vi "02Config_equipos.vi"(4 "EE 568 M IN":T2(array[cluster]) {"Analogicas 32"."?" items=["1", "2", "4", "8", "16", "32", "64", "128", "256"]; "Analogicas 32"."?" items=["Lineal"=15, "Cuadrática"=14]; "Analogicas 32"."unsigned byte array[0]" items=["10000", "1000", "100", "10", "8000", "800", "80", "8", "4000", "400", "40", "4", "2000", "200", "20", "2"]; "Analogicas 16"."?" items=["1", "2", "4", "8", "16", "32", "64", "128", "256"]; "Analogicas 16"."?" items=["Lineal"=15, "Cuadrática"=14]; "Analogicas 16"."unsigned byte array[0]" items=["10000", "1000", "100", "10", "8000", "800", "80", "8", "4000", "400", "40", "4", "2000", "200", "20", "2"]}, 6 "Equipo Nº":i32(ring) caption="PANEL DE EQUIPO\nA CONFIGURAR" items=["1", "2", "3", "4", "5", "6", "7", "8", "9", "10", "11", "12", "13", "14", "15", "16", "17", "18", "19", "20", "21", "22", "23", "24", "25"], 7 "EE 568 S IN":T2(array[cluster]) {"Analogicas 32"."?" items=["1", "2", "4", "8", "16", "32", "64", "128", "256"]; "Analogicas 32"."?" items=["Lineal"=15, "Cuadrática"=14]; "Analogicas 32"."unsigned byte array[0]" items=["10000", "1000", "100", "10", "8000", "800", "80", "8", "4000", "400", "40", "4", "2000", "200", "20", "2"]; "Analogicas 16"."?" items=["1", "2", "4", "8", "16", "32", "64", "128", "256"]; "Analogicas 16"."?" items=["Lineal"=15, "Cuadrática"=14]; "Analogicas 16"."unsigned byte array[0]" items=["10000", "1000", "100", "10", "8000", "800", "80", "8", "4000", "400", "40", "4", "2000", "200", "20", "2"]}, 8 "Paneles in":T4(array[cluster]) {"Nº" min=1.0 max=60.0 step=1.0 format="%#2.1f"; "Ultima recepción" format="%<%d/%m - %X>T"; "Med\nPpal" format="%_4g"}, 9 "Config Equipos ent":T6(array[cluster]) {"Ref PD 2" max=10000 step=1; "Med Princ" items=["1", "2", "3", "4", "5", "6", "7", "8", "9", "10", "11", "12", "13", "14", "15", "16", "17", "18", "19", "20", "21", "22", "23", "24", "25", "26", "27", "28", "29", "30", "31", "32"]}, 10 "EE 492 in":T5(array[cluster]), 11 "Exe path":string) -> (0 "Paneles out":T3(array[cluster]) {"Numeric" min=1.0 max=60.0 step=1.0 format="%#2.1f"; "Ultima recepción" format="%<%d/%m - %X>T"; "Med\nPpal" format="%_4g"}, 1 "EE 568 M OUT":T2(array[cluster]) {"Analogicas 32"."?" items=["1", "2", "4", "8", "16", "32", "64", "128", "256"]; "Analogicas 32"."?" items=["Lineal"=15, "Cuadrática"=14]; "Analogicas 32"."unsigned byte array[0]" items=["10000", "1000", "100", "10", "8000", "800", "80", "8", "4000", "400", "40", "4", "2000", "200", "20", "2"]; "Analogicas 16"."?" items=["1", "2", "4", "8", "16", "32", "64", "128", "256"]; "Analogicas 16"."?" items=["Lineal"=15, "Cuadrática"=14]; "Analogicas 16"."unsigned byte array[0]" items=["10000", "1000", "100", "10", "8000", "800", "80", "8", "4000", "400", "40", "4", "2000", "200", "20", "2"]}, 2 "Config Equipos sal":T6(array[cluster]) {"Ref PD 2" max=10000 step=1; "Med Princ" items=["1", "2", "3", "4", "5", "6", "7", "8", "9", "10", "11", "12", "13", "14", "15", "16", "17", "18", "19", "20", "21", "22", "23", "24", "25", "26", "27", "28", "29", "30", "31", "32"]}, 3 "EE 492 OUT":T5(array[cluster]), 5 "EE 568 S OUT":T2(array[cluster]) {"Analogicas 32"."?" items=["1", "2", "4", "8", "16", "32", "64", "128", "256"]; "Analogicas 32"."?" items=["Lineal"=15, "Cuadrática"=14]; "Analogicas 32"."unsigned byte array[0]" items=["10000", "1000", "100", "10", "8000", "800", "80", "8", "4000", "400", "40", "4", "2000", "200", "20", "2"]; "Analogicas 16"."?" items=["1", "2", "4", "8", "16", "32", "64", "128", "256"]; "Analogicas 16"."?" items=["Lineal"=15, "Cuadrática"=14]; "Analogicas 16"."unsigned byte array[0]" items=["10000", "1000", "100", "10", "8000", "800", "80", "8", "4000", "400", "40", "4", "2000", "200", "20", "2"]})   [LabVIEW 2010]
uses:
  <vilib>/Utility/error.llb/whitespace.ctl
panel:
  out "eeprom re-cod":string
  out "Eeprom D-cod M":T1={"Rotulo 1"="TRUD1200", "Rotulo 2"="     PD SALIDA [Wrms]  ", "Cant. Meds."=32, "Med ampl"=0, "Analogicas 16"=[{"Nº"=1, "Nombre"="PD_SAL ", "Unidad"=" W ", 14, "unsigned byte array[0]"=12, 5}, {"Nº"=2, "Nombre"="PR_SAL ", "Unidad"=" W ", 14, "unsigned byte array[0]"=9, 5}, {"Nº"=3, "Nombre"="PD_AMP1", "Unidad"=" W ", 14, "unsigned byte array[0]"=9, 4}, {"Nº"=4, "Nombre"="PD_AMP2", "Unidad"=" W ", 14, "unsigned byte array[0]"=9, 4}, {"Nº"=5, "Nombre"="PD_AMP3", "Unidad"=" W ", 14, "unsigned byte array[0]"=9, 4}, {"Nº"=6, "Nombre"="PD_AMP4", "Unidad"=" W ", 14, "unsigned byte array[0]"=9, 4}, {"Nº"=7, "Nombre"="PD_AMP5", "Unidad"=" W ", 14, "unsigned byte array[0]"=9, 4}, {"Nº"=8, "Nombre"="PD_AMP6", "Unidad"=" W ", 14, "unsigned byte array[0]"=9, 4}, {"Nº"=9, "Nombre"="V_AMP1 ", "Unidad"=" V ", 15, "unsigned byte array[0]"=6, 4}, {"Nº"=10, "Nombre"="I_AMP1 ", "Unidad"=" A ", 15, "unsigned byte array[0]"=10, 4}, {"Nº"=11, "Nombre"="V_AMP2 ", "Unidad"=" V ", 15, "unsigned byte array[0]"=6, 4}, {"Nº"=12, "Nombre"="I_AMP2 ", "Unidad"=" A ", 15, "unsigned byte array[0]"=10, 4}, {"Nº"=13, "Nombre"="V_AMP3 ", "Unidad"=" V ", 15, "unsigned byte array[0]"=6, 4}, {"Nº"=14, "Nombre"="I_AMP3 ", "Unidad"=" A ", 15, "unsigned byte array[0]"=10, 4}, {"Nº"=15, "Nombre"="V_AMP4 ", "Unidad"=" V ", 15, "unsigned byte array[0]"=6, 4}, {"Nº"=16, "Nombre"="I_AMP4 ", "Unidad"=" A ", 15, "unsigned byte array[0]"=10, 4}], "Analogicas 32"=[{17, "mapaeeprom"="V_AMP5 ", "mapaeeprom"=" V ", 15, "unsigned byte array[0]"=6, 4}, {18, "mapaeeprom"="I_AMP5 ", "mapaeeprom"=" A ", 15, "unsigned byte array[0]"=10, 4}, {19, "mapaeeprom"="V_AMP6 ", "mapaeeprom"=" V ", 15, "unsigned byte array[0]"=6, 4}, {20, "mapaeeprom"="I_AMP6 ", "mapaeeprom"=" A ", 15, "unsigned byte array[0]"=10, 4}, {21, "mapaeeprom"="VL_1   ", "mapaeeprom"="Vca", 15, "unsigned byte array[0]"=9, 5}, {22, "mapaeeprom"="VL_2   ", "mapaeeprom"="Vca", 15, "unsigned byte array[0]"=9, 5}, {23, "mapaeeprom"="VL_3   ", "mapaeeprom"="Vca", 15, "unsigned byte array[0]"=9, 5}, {24, "mapaeeprom"="T_CTRL ", "mapaeeprom"=" *C", 15, "unsigned byte array[0]"=2, 5}, {25, "mapaeeprom"="P_EXC_1", "mapaeeprom"=" W ", 14, "unsigned byte array[0]"=10, 5}, {26, "mapaeeprom"="I_EXC_1", "mapaeeprom"=" A ", 15, "unsigned byte array[0]"=10, 4}, {27, "mapaeeprom"="SET_P_1", "mapaeeprom"="/63", 15, "unsigned byte array[0]"=2, 4}, {28, "mapaeeprom"="P_MOD_1", "mapaeeprom"=" mW", 14, "unsigned byte array[0]"=10, 5}, {29, "mapaeeprom"="P_EXC_2", "mapaeeprom"=" W ", 14, "unsigned byte array[0]"=10, 5}, {30, "mapaeeprom"="I_EXC_2", "mapaeeprom"=" A ", 15, "unsigned byte array[0]"=10, 4}, {31, "mapaeeprom"="SET_P_2", "mapaeeprom"="/63", 15, "unsigned byte array[0]"=2, 4}, {32, "mapaeeprom"="P_MOD_2", "mapaeeprom"=" mW", 14, "unsigned byte array[0]"=10, 5}], "DIG_8"=[{"ESTADO"=TRUE, "VAL_INI"=TRUE, "VAL_FIJO"=FALSE, "VAL_CORTE"=FALSE, "Nombre"="0E_TXE2"}, {"ESTADO"=TRUE, "VAL_INI"=TRUE, "VAL_FIJO"=FALSE, "VAL_CORTE"=FALSE, "Nombre"="1E_RVOF"}, {"ESTADO"=TRUE, "VAL_INI"=TRUE, "VAL_FIJO"=FALSE, "VAL_CORTE"=FALSE, "Nombre"="2E_SN1 "}, {"ESTADO"=TRUE, "VAL_INI"=TRUE, "VAL_FIJO"=FALSE, "VAL_CORTE"=FALSE, "Nombre"="3E_SN2 "}, {"ESTADO"=TRUE, "VAL_INI"=TRUE, "VAL_FIJO"=FALSE, "VAL_CORTE"=FALSE, "Nombre"="4E_SN3 "}, {"ESTADO"=TRUE, "VAL_INI"=TRUE, "VAL_FIJO"=FALSE, "VAL_CORTE"=FALSE, "Nombre"="5E_SN4 "}, {"ESTADO"=FALSE, "VAL_INI"=TRUE, "VAL_FIJO"=FALSE, "VAL_CORTE"=FALSE, "Nombre"="6S_CMT1"}, {"ESTADO"=FALSE, "VAL_INI"=TRUE, "VAL_FIJO"=FALSE, "VAL_CORTE"=FALSE, "Nombre"="7S_CMT2"}], "DIG_16"=[{"ESTADO"=FALSE, "VAL_INI"=FALSE, "VAL_FIJO"=FALSE, "VAL_CORTE"=FALSE, "Nombre"="8S_CMS1"}, {"ESTADO"=FALSE, "VAL_INI"=FALSE, "VAL_FIJO"=FALSE, "VAL_CORTE"=FALSE, "Nombre"="9S_CMS2"}, {"ESTADO"=FALSE, "VAL_INI"=TRUE, "VAL_FIJO"=FALSE, "VAL_CORTE"=FALSE, "Nombre"="AS_CMT3"}, {"ESTADO"=TRUE, "VAL_INI"=TRUE, "VAL_FIJO"=FALSE, "VAL_CORTE"=FALSE, "Nombre"="BE_REM "}, {"ESTADO"=TRUE, "VAL_INI"=TRUE, "VAL_FIJO"=FALSE, "VAL_CORTE"=FALSE, "Nombre"="CE_M>R "}, {"ESTADO"=TRUE, "VAL_INI"=TRUE, "VAL_FIJO"=FALSE, "VAL_CORTE"=FALSE, "Nombre"="DE_POK "}, {"ESTADO"=TRUE, "VAL_INI"=TRUE, "VAL_FIJO"=FALSE, "VAL_CORTE"=FALSE, "Nombre"="EE_LOA "}, {"ESTADO"=TRUE, "VAL_INI"=TRUE, "VAL_FIJO"=FALSE, "VAL_CORTE"=FALSE, "Nombre"="FE_<RV "}], "PWM"={"CONF_PWM1"=255, "VALOR_PWM1"=255, "CONF_PWM2"=255, "VALOR_PWM2"=255}} {"Analogicas 32"."?" items=["1", "2", "4", "8", "16", "32", "64", "128", "256"]; "Analogicas 32"."?" items=["Lineal"=15, "Cuadrática"=14]; "Analogicas 32"."unsigned byte array[0]" items=["10000", "1000", "100", "10", "8000", "800", "80", "8", "4000", "400", "40", "4", "2000", "200", "20", "2"]; "Analogicas 16"."?" items=["1", "2", "4", "8", "16", "32", "64", "128", "256"]; "Analogicas 16"."?" items=["Lineal"=15, "Cuadrática"=14]; "Analogicas 16"."unsigned byte array[0]" items=["10000", "1000", "100", "10", "8000", "800", "80", "8", "4000", "400", "40", "4", "2000", "200", "20", "2"]}
  out "Eeprom D-cod S":T1={"Rotulo 1"="Med33-64", "Rotulo 2"=" T_SUMADOR [C]         ", "Cant. Meds."=32, "Med ampl"=17, "Analogicas 16"=[{"Nº"=1, "Nombre"="PR_AMP1", "Unidad"=" W ", 14, "unsigned byte array[0]"=6, 4}, {"Nº"=2, "Nombre"="T_AMP_1", "Unidad"=" *C", 15, "unsigned byte array[0]"=2, 4}, {"Nº"=3, "Nombre"="PR_AMP2", "Unidad"=" W ", 14, "unsigned byte array[0]"=6, 4}, {"Nº"=4, "Nombre"="T_AMP_2", "Unidad"=" *C", 15, "unsigned byte array[0]"=2, 4}, {"Nº"=5, "Nombre"="PR_AMP3", "Unidad"=" W ", 14, "unsigned byte array[0]"=6, 4}, {"Nº"=6, "Nombre"="T_AMP_3", "Unidad"=" *C", 15, "unsigned byte array[0]"=2, 4}, {"Nº"=7, "Nombre"="PR_AMP4", "Unidad"=" W ", 14, "unsigned byte array[0]"=6, 4}, {"Nº"=8, "Nombre"="T_AMP_4", "Unidad"=" *C", 15, "unsigned byte array[0]"=2, 4}, {"Nº"=9, "Nombre"="PR_AMP5", "Unidad"=" W ", 14, "unsigned byte array[0]"=6, 4}, {"Nº"=10, "Nombre"="T_AMP_5", "Unidad"=" *C", 15, "unsigned byte array[0]"=2, 4}, {"Nº"=11, "Nombre"="PR_AMP6", "Unidad"=" W ", 14, "unsigned byte array[0]"=6, 4}, {"Nº"=12, "Nombre"="T_AMP_6", "Unidad"=" *C", 15, "unsigned byte array[0]"=2, 4}, {"Nº"=13, "Nombre"="V_EXC_1", "Unidad"=" V ", 15, "unsigned byte array[0]"=6, 4}, {"Nº"=14, "Nombre"="V_CAG_1", "Unidad"=" V ", 15, "unsigned byte array[0]"=14, 4}, {"Nº"=15, "Nombre"="V_EXC_2", "Unidad"=" V ", 15, "unsigned byte array[0]"=6, 4}, {"Nº"=16, "Nombre"="V_CAG_2", "Unidad"=" V ", 15, "unsigned byte array[0]"=14, 4}], "Analogicas 32"=[{17, "mapaeeprom"="V_AUX  ", "mapaeeprom"=" V ", 15, "unsigned byte array[0]"=14, 4}, {18, "mapaeeprom"="T_SUM  ", "mapaeeprom"=" *C", 15, "unsigned byte array[0]"=2, 4}, {19, "mapaeeprom"="T_EXC_1", "mapaeeprom"=" *C", 15, "unsigned byte array[0]"=2, 4}, {20, "mapaeeprom"="T_EXC_2", "mapaeeprom"=" *C", 15, "unsigned byte array[0]"=2, 4}, {21, "mapaeeprom"="V_EXT_1", "mapaeeprom"=" V ", 15, "unsigned byte array[0]"=14, 4}, {22, "mapaeeprom"="V_EXT_2", "mapaeeprom"=" V ", 15, "unsigned byte array[0]"=14, 4}, {23, "mapaeeprom"="V_EXT_3", "mapaeeprom"=" V ", 15, "unsigned byte array[0]"=14, 4}, {24, "mapaeeprom"="V_EXT_4", "mapaeeprom"=" V ", 15, "unsigned byte array[0]"=14, 4}, {25, "mapaeeprom"="V_EXT_5", "mapaeeprom"=" V ", 15, "unsigned byte array[0]"=14, 4}, {26, "mapaeeprom"="V_EXT_6", "mapaeeprom"=" V ", 15, "unsigned byte array[0]"=14, 4}, {27, "mapaeeprom"="V_EXT_7", "mapaeeprom"=" V ", 15, "unsigned byte array[0]"=14, 4}, {28, "mapaeeprom"="V_EXT_8", "mapaeeprom"=" V ", 15, "unsigned byte array[0]"=14, 4}, {29, "mapaeeprom"="V_EXT_9", "mapaeeprom"=" V ", 15, "unsigned byte array[0]"=14, 4}, {30, "mapaeeprom"="V_EXT10", "mapaeeprom"=" V ", 15, "unsigned byte array[0]"=14, 4}, {31, "mapaeeprom"="V_EXT11", "mapaeeprom"=" V ", 15, "unsigned byte array[0]"=14, 4}, {32, "mapaeeprom"="V_EXT12", "mapaeeprom"=" V ", 15, "unsigned byte array[0]"=14, 4}], "DIG_8"=[{"ESTADO"=TRUE, "VAL_INI"=TRUE, "VAL_FIJO"=FALSE, "VAL_CORTE"=FALSE, "Nombre"="GE_INX1"}, {"ESTADO"=TRUE, "VAL_INI"=TRUE, "VAL_FIJO"=FALSE, "VAL_CORTE"=FALSE, "Nombre"="HE_INX2"}, {"ESTADO"=TRUE, "VAL_INI"=TRUE, "VAL_FIJO"=FALSE, "VAL_CORTE"=FALSE, "Nombre"="IE_INX3"}, {"ESTADO"=TRUE, "VAL_INI"=TRUE, "VAL_FIJO"=FALSE, "VAL_CORTE"=FALSE, "Nombre"="JE_INX4"}, {"ESTADO"=TRUE, "VAL_INI"=TRUE, "VAL_FIJO"=FALSE, "VAL_CORTE"=FALSE, "Nombre"="KE_INX5"}, {"ESTADO"=TRUE, "VAL_INI"=TRUE, "VAL_FIJO"=FALSE, "VAL_CORTE"=FALSE, "Nombre"="LE_INX6"}, {"ESTADO"=TRUE, "VAL_INI"=TRUE, "VAL_FIJO"=FALSE, "VAL_CORTE"=FALSE, "Nombre"="ME_INX7"}, {"ESTADO"=TRUE, "VAL_INI"=TRUE, "VAL_FIJO"=FALSE, "VAL_CORTE"=FALSE, "Nombre"="NE_INX8"}], "DIG_16"=[{"ESTADO"=FALSE, "VAL_INI"=FALSE, "VAL_FIJO"=FALSE, "VAL_CORTE"=FALSE, "Nombre"="PS_CMX1"}, {"ESTADO"=FALSE, "VAL_INI"=FALSE, "VAL_FIJO"=FALSE, "VAL_CORTE"=FALSE, "Nombre"="QS_CMX2"}, {"ESTADO"=FALSE, "VAL_INI"=FALSE, "VAL_FIJO"=FALSE, "VAL_CORTE"=FALSE, "Nombre"="RS_CMX3"}, {"ESTADO"=FALSE, "VAL_INI"=FALSE, "VAL_FIJO"=FALSE, "VAL_CORTE"=FALSE, "Nombre"="SS_CMX4"}, {"ESTADO"=FALSE, "VAL_INI"=FALSE, "VAL_FIJO"=FALSE, "VAL_CORTE"=FALSE, "Nombre"="TS_CMX5"}, {"ESTADO"=FALSE, "VAL_INI"=FALSE, "VAL_FIJO"=FALSE, "VAL_CORTE"=FALSE, "Nombre"="US_CMX6"}, {"ESTADO"=FALSE, "VAL_INI"=FALSE, "VAL_FIJO"=FALSE, "VAL_CORTE"=FALSE, "Nombre"="VS_CMX7"}, {"ESTADO"=FALSE, "VAL_INI"=FALSE, "VAL_FIJO"=FALSE, "VAL_CORTE"=FALSE, "Nombre"="WS_CMX8"}], "PWM"={"CONF_PWM1"=255, "VALOR_PWM1"=255, "CONF_PWM2"=255, "VALOR_PWM2"=255}} {"Analogicas 32"."?" items=["1", "2", "4", "8", "16", "32", "64", "128", "256"]; "Analogicas 32"."?" items=["Lineal"=15, "Cuadrática"=14]; "Analogicas 32"."unsigned byte array[0]" items=["10000", "1000", "100", "10", "8000", "800", "80", "8", "4000", "400", "40", "4", "2000", "200", "20", "2"]; "Analogicas 16"."?" items=["1", "2", "4", "8", "16", "32", "64", "128", "256"]; "Analogicas 16"."?" items=["Lineal"=15, "Cuadrática"=14]; "Analogicas 16"."unsigned byte array[0]" items=["10000", "1000", "100", "10", "8000", "800", "80", "8", "4000", "400", "40", "4", "2000", "200", "20", "2"]}
  out "error out":errorcluster
  out "Config equipo":T7={"Modelo"="", "IP "="", "Puerto:"=0, "Time Out"=0, "Med Princ"=0, "Time sin rx"=60, "Reintento"=0, "Ref PD"=200} {"Ref PD" max=10000 step=1}
  in  "Flag write":bool=TRUE
  in  "CODIGO":string
  out "Pagina 2":string
  out "Pagina 1":string
  out "nPAG2":u8
  out "nPAG1":u8
  in  "ARRAY 2":T8(array[cluster])
  in  "ARRAY 1":T8(array[cluster])
  in  "Mapa Ee 492":string
  in  "Tab\nControl":T9(tab)
  in  "Destino":u16=2 caption="Panel Nº" min=1 max=100 step=1
  in  "<<-------->>":bool
  in  "Origen":u16=1 caption="Panel Nº" min=1 max=100 step=1
  in  "Ref PD":u16=20 caption="Referencia potencia baja\nPD [W]" max=10000 step=1
  in  "Config avanz":bool
  in  "Guardar":bool
  in  "Cargar":bool
  in  "Nombre:":string caption="Nombre Equipo:"
  in  "Puerto:":u16=2101 caption="Puerto [2101]:"
  in  "IP":string(combo)="192.168.0.200" caption="Dirección IP (o DNS name)"
  in  "Med Princ":u16(ring) caption="Medicion Principal" items=["1", "2", "3", "4", "5", "6", "7", "8", "9", "10", "11", "12", "13", "14", "15", "16", "17", "18", "19", "20", "21", "22", "23", "24", "25", "26", "27", "28", "29", "30", "31", "32"]
  in  "Time Out":u16=500 caption="Time Out [ms]" min=100 max=25000 step=50
  in  "Reintento":u16=60 caption="Reintentar\nconexion [s]"
  in  "Modelo":string(combo)="TRV100"
  in  "Conexion\n Placa":bool caption="Conexion?"
  out "Tx test":string
  out "Rx test":string
  in  "Time sin rx":u16=20 caption="Tiempo aviso\nsin RX [s]"
  in  "Stop":bool
  out "Tab placa":enum32{"492", "568"}(tab)
  in  "Menu 492:":u16(ring) caption="Manejo de datos:" items=["   Menu:"=0, "_______________"=101, "Abrir Archivo"=1, "Guardar Como..."=2, "_______________"=102, "Leer Memoria"=3, "Grabar Memoria"=4, "_______________"=103, "Reset Panel"=6, "_______________"=104, "Salir"=5]
  in  "Recuperar":bool
  out "Recup?":bool=TRUE
  in  "Med 1-4":T10(array[cluster]) {"?" items=["1", "2", "4", "8", "16", "32", "64", "128", "256"]; "?" items=["Tabla"=2.0, "Lineal"=15.0, "Cuadrática"=14.0]; "unsigned byte array[0]" items=["1"=3, "2"=7, "4"=11, "10"=2, "20"=6, "40"=10, "100"=1, "200"=5, "400"=9, "1000"=0, "2000"=4, "4000"=8]}
  in  "Med 9-12":T10(array[cluster]) {"?" items=["1", "2", "4", "8", "16", "32", "64", "128", "256"]; "?" items=["Tabla"=2.0, "Lineal"=15.0, "Cuadrática"=14.0]; "unsigned byte array[0]" items=["1"=3, "2"=7, "4"=11, "10"=2, "20"=6, "40"=10, "100"=1, "200"=5, "400"=9, "1000"=0, "2000"=4, "4000"=8]}
  in  "Med 13-16":T10(array[cluster]) {"?" items=["1", "2", "4", "8", "16", "32", "64", "128", "256"]; "?" items=["Tabla"=2.0, "Lineal"=15.0, "Cuadrática"=14.0]; "unsigned byte array[0]" items=["1"=3, "2"=7, "4"=11, "10"=2, "20"=6, "40"=10, "100"=1, "200"=5, "400"=9, "1000"=0, "2000"=4, "4000"=8]}
  in  "Med 17-20":T10(array[cluster]) {"?" items=["1", "2", "4", "8", "16", "32", "64", "128", "256"]; "?" items=["Tabla"=2.0, "Lineal"=15.0, "Cuadrática"=14.0]; "unsigned byte array[0]" items=["1"=3, "2"=7, "4"=11, "10"=2, "20"=6, "40"=10, "100"=1, "200"=5, "400"=9, "1000"=0, "2000"=4, "4000"=8]}
  in  "Med 21-24":T10(array[cluster]) {"?" items=["1", "2", "4", "8", "16", "32", "64", "128", "256"]; "?" items=["Tabla"=2.0, "Lineal"=15.0, "Cuadrática"=14.0]; "unsigned byte array[0]" items=["1"=3, "2"=7, "4"=11, "10"=2, "20"=6, "40"=10, "100"=1, "200"=5, "400"=9, "1000"=0, "2000"=4, "4000"=8]}
  in  "Med 25-28":T10(array[cluster]) {"?" items=["1", "2", "4", "8", "16", "32", "64", "128", "256"]; "?" items=["Tabla"=2.0, "Lineal"=15.0, "Cuadrática"=14.0]; "unsigned byte array[0]" items=["1"=3, "2"=7, "4"=11, "10"=2, "20"=6, "40"=10, "100"=1, "200"=5, "400"=9, "1000"=0, "2000"=4, "4000"=8]}
  in  "Med 5-8":T10(array[cluster]) {"?" items=["1", "2", "4", "8", "16", "32", "64", "128", "256"]; "?" items=["Tabla"=2.0, "Lineal"=15.0, "Cuadrática"=14.0]; "unsigned byte array[0]" items=["1"=3, "2"=7, "4"=11, "10"=2, "20"=6, "40"=10, "100"=1, "200"=5, "400"=9, "1000"=0, "2000"=4, "4000"=8]}
  in  "Señales Logicas:":cluster{i32, "mapaeeprom":string, bool}[][](array[cluster])
  out "Nom Med Ampl":string
  in  "Medición Ampliada:":u8(ring) items=["1", "2", "3", "4", "5", "6", "7", "8", "9", "10", "11", "12", "13", "14", "15", "16", "17", "18", "19", "20", "21", "22", "23", "24", "25", "26", "27", "28", "29", "30", "31", "32"]
  in  "Cant Med:":u8(ring) items=["4"=4, "8"=8, "12"=12, "16"=16, "20"=20, "24"=24, "28"=28, "32"=32]
  in  "Rotulo izquierdo:":string
  in  "Rotulo derecho:":string
  in  "Med 29-32":T10(array[cluster]) {"?" items=["1", "2", "4", "8", "16", "32", "64", "128", "256"]; "?" items=["Tabla"=2.0, "Lineal"=15.0, "Cuadrática"=14.0]; "unsigned byte array[0]" items=["1"=3, "2"=7, "4"=11, "10"=2, "20"=6, "40"=10, "100"=1, "200"=5, "400"=9, "1000"=0, "2000"=4, "4000"=8]}
  out "Menu light":bool=TRUE caption="hola"
  in  "Menu 568:":u8(ring) caption="Manejo de datos:" items=["   Menu:"=0, "_______________"=101, "Abrir Archivo"=1, "Guardar Como..."=2, "_______________"=102, "Leer Memoria"=3, "Grabar Memoria"=4, "_______________"=103, "Reset Panel"=6, "_______________"=104, "Salir"=5]
  out "Menu light 2":bool=TRUE caption="hola"
  in  "Ana 32":T11(array[cluster]) {"Promediacion" items=["1", "4", "8", "16", "32", "64", "128", "256"]; "Linealidad" items=["Cuadrática"=14, "Lineal"=15]; "Escala" items=["2"=15, "4"=11, "8"=7, "10"=3, "20"=14, "40"=10, "80"=6, "100"=2, "200"=13, "400"=9, "800"=5, "1.000"=1, "2.000"=12, "4.000"=8, "8.000"=4, "10.000"=0]}
  in  "PWM data 1&2":T12
  in  "DIG_16":T13(array[cluster]) caption="SEÑALES\nLOGICAS\n L9-L16"
  in  "DIG_8":T13(array[cluster]) caption="SEÑALES\nLOGICAS\n L1-L8"
  in  "Ana 16":T11(array[cluster]) {"Promediacion" items=["1", "4", "8", "16", "32", "64", "128", "256"]; "Linealidad" items=["Cuadrática"=14, "Lineal"=15]; "Escala" items=["2"=15, "4"=11, "8"=7, "10"=3, "20"=14, "40"=10, "80"=6, "100"=2, "200"=13, "400"=9, "800"=5, "1.000"=1, "2.000"=12, "4.000"=8, "8.000"=4, "10.000"=0]}
  in  "Medición Ampliada: 2":u8(ring) caption="Medición\nAmpliada" items=["1", "2", "3", "4", "5", "6", "7", "8", "9", "10", "11", "12", "13", "14", "15", "16", "17", "18", "19", "20", "21", "22", "23", "24", "25", "26", "27", "28", "29", "30", "31", "32"]
  in  "Cantidad\nMediciones":u8(ring) items=["0"=0, "4"=4, "8"=8, "12"=12, "16"=16, "20"=20, "24"=24, "28"=28, "32"=32]
  in  "Título Secundario:":string
  in  "Título Principal:":string
  out "COMFAIL M":bool caption="COM\nFAIL"
  in  "MASTER\n/SLAVE":bool
  in  "Slave Nº":u8(ring)=3 items=["Slave Nº 03"=3, "Slave Nº 05"=5, "Slave Nº 07"=7, "Slave Nº 09"=9, "Slave Nº 11"=11, "Slave Nº 13"=13, "Slave Nº 15"=15]
  # "CONFIGURACIÓN DE EQUIPOS"
  # "Telemedición XME"
  # "Configuración del equipo:"
  # "Configuración de conexión:"
  # "Intercambiar Configs."
  # "Transmisión:"
  # "Recepción:"
  # "SEÑALES ANALÓGICAS 1-16:"
  # "SEÑALES ANALÓGICAS 17-32:"
  # "Nº"
  # "Nombre"
  # "Unidad"
  # "Tipo"
  # "F. Escala"
  # "Promediar"
  # "Nº"
  # "Nombre"
  # "Unidad"
  # "Tipo"
  # "F. Escala"
  # "Promediar"
  # "SEÑALES LOGICAS:"
  # "Nº"
  # "Nombre"
  # "IN/OUT"
  # "CONTROL DATOS"
  # "SEÑALES ANALÓGICAS A1-A16:"
  # "SEÑALES ANALÓGICAS A17-A32:"
  # "Nº"
  # "Nombre"
  # "Unidad"
  # "Tipo"
  # "F. Escala"
  # "Promediar"
  # "Nº"
  # "Nombre"
  # "Unidad"
  # "Tipo"
  # "F. Escala"
  # "Promediar"
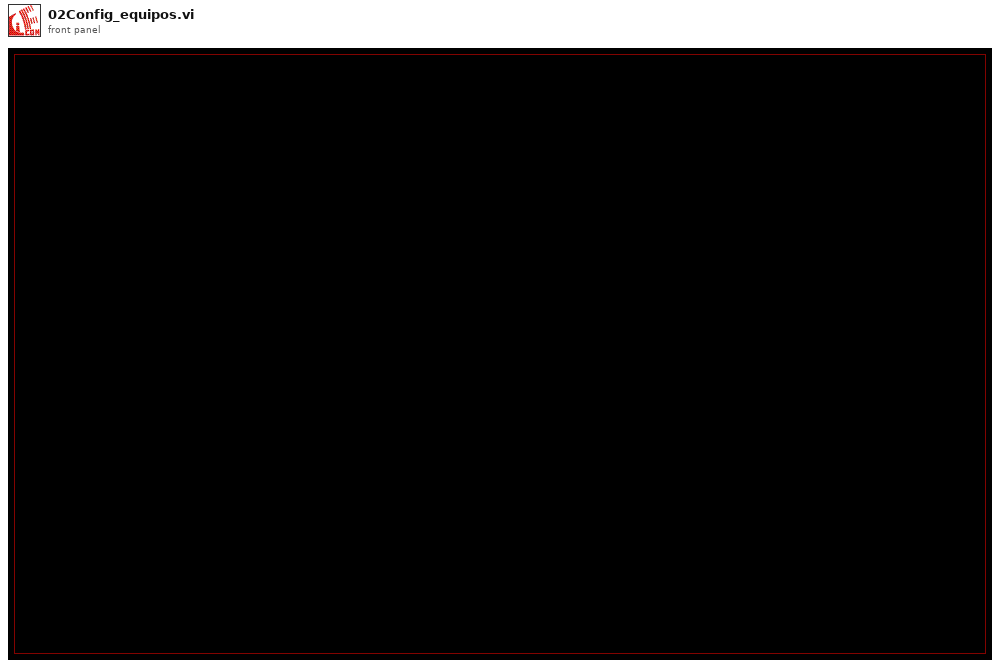
[diagram p1: front panel]
types:
  T1 = cluster{"Rotulo 1":string, "Rotulo 2":string, "Cant. Meds.":u8, "Med ampl":u8, "Analogicas 16":cluster{"Nº":i32, "Nombre":string, "Unidad":string, u8, "unsigned byte array[0]":u8, u8}[], "Analogicas 32":cluster{i32, "mapaeeprom":string, "mapaeeprom":string, u8, "unsigned byte array[0]":u8, u8}[], "DIG_8":cluster{"ESTADO":bool, "VAL_INI":bool, "VAL_FIJO":bool, "VAL_CORTE":bool, "Nombre":string}[], "DIG_16":cluster{"ESTADO":bool, "VAL_INI":bool, "VAL_FIJO":bool, "VAL_CORTE":bool, "Nombre":string}[], "PWM":cluster{"CONF_PWM1":u8, "VALOR_PWM1":u8, "CONF_PWM2":u8, "VALOR_PWM2":u8}}
  T2 = cluster{"Rotulo 1":string, "Rotulo 2":string, "Cant. Meds.":u8, "Med ampl":u8, "Analogicas 16":cluster{"Nº":i32, "Nombre":string, "Unidad":string, u8, "unsigned byte array[0]":u8, u8}[], "Analogicas 32":cluster{i32, "mapaeeprom":string, "mapaeeprom":string, u8, "unsigned byte array[0]":u8, u8}[], "DIG_8":cluster{"ESTADO":bool, "VAL_INI":bool, "VAL_FIJO":bool, "VAL_CORTE":bool, "Nombre":string}[], "DIG_16":cluster{"ESTADO":bool, "VAL_INI":bool, "VAL_FIJO":bool, "VAL_CORTE":bool, "Nombre":string}[], "PWM":cluster{"CONF_PWM1":u8, "VALOR_PWM1":u8, "CONF_PWM2":u8, "VALOR_PWM2":u8}}[]
  T3 = cluster{"Nombre":string, "Med\nPpal":dbl, "On/Off":bool, "Ultima recepción":timestamp, "Numeric":dbl, "deshabilitacion":bool, "Prioridad":bool, "falla":bool, "alarm":bool}[][]
  T4 = cluster{"Nombre":string, "Med\nPpal":dbl, "On/Off":bool, "Ultima recepción":timestamp, "Nº":dbl, "deshabilitacion":bool, "Prioridad":bool, "falla":bool, "alarm":bool}[][]
  T5 = cluster{"mapaeeprom":string, "cantmedic":u8, "Med_nom":string[], "Med_unid":string[], "Med_caract":string}[]
  T6 = cluster{"Modelo":string, "IP":string, "Puerto":u16, "Time Out":u16, "Med Princ":u16, "Time sin rx":u16, "Reintento":u16, "Ref PD 2":u16}[]
  T7 = cluster{"Modelo":string, "IP ":string, "Puerto:":u16, "Time Out":u16, "Med Princ":u16, "Time sin rx":u16, "Reintento":u16, "Ref PD":u16}
  T8 = cluster{i32, "mapaeeprom":string, "mapaeeprom":string, dbl, u8, "unsigned byte array[0]":u8}[][]
  T9 = enum32{"Configuración Equipo", "Configuración Placa"}
  T10 = cluster{i32, "mapaeeprom":string, "mapaeeprom":string, dbl, "unsigned byte array[0]":u8, u8}[][]
  T11 = cluster{"Nº":i32, "Nombre":string, "Unidad":string, "Linealidad":u8, "Escala":u8, "Promediacion":u8}[]
  T12 = cluster{"CONFIG\nPWM1":u8, "VALOR\nPWM1":u8, "CONFIG\nPWM2":u8, "VALOR\nPWM2":u8}
  T13 = cluster{"ESTADO":bool, "VAL_INI":bool, "VAL_FIJO":bool, "VAL_CORTE":bool, "Nombre":string}[]
  T14 = enum32{"Configuración Equipo", "Configuración Placa", "inicio"}
  T15 = cluster{"CONF_PWM1":u8, "VALOR_PWM1":u8, "CONF_PWM2":u8, "VALOR_PWM2":u8}
  T16 = cluster{"Nombre":string, "Med\nprinc":dbl, "On/Off":bool, "Ultima recepción":timestamp, "Nº":dbl, "deshabilitacion":bool, "Actividad":bool, "falla":bool, "alarm":bool}
  T17 = cluster{"Modelo":string, "IP":string, "Puerto":u16, "Time Out":u16, "Med Princ":u16, "Time sin rx":u16, "Reintento":u16, "Ref PD 2":u16}
  T18 = cluster{"Modelo":string, "IP":string, "Puerto:":u16, "Time Out":u16, "Med Princ":u16, "Time sin rx":u16, "Reintento":u16, "Ref PD":u16}
  T19 = cluster{"Nombre:":string, "Med\nprinc":dbl, "On/Off":bool, "Ultima recepción":timestamp, "Nº":dbl, "deshabilitacion":bool, "Actividad":bool, "falla":bool, "alarm":bool}
  T20 = cluster{"Nombre":string, "Med\nPpal":dbl, "On/Off":bool, "Ultima recepción":timestamp, "Numeric":dbl, "deshabilitacion":bool, "Prioridad 2":bool, "falla":bool, "alarm":bool}[][]
  T21 = typedef "whitespace.ctl" = u16
  T22 = cluster{i32, "mapaeeprom":string, "mapaeeprom":string, dbl, u8, "unsigned byte array[0]":u8}[]
  T23 = cluster{"ARRAY 2[0]":cluster{i32, "mapaeeprom":string, "mapaeeprom":string, dbl, u8, "unsigned byte array[0]":u8}}
  T24 = cluster{i32, "mapaeeprom":string, "mapaeeprom":string, dbl, u8, "unsigned byte array[0]":u8}
  T25 = cluster{"ARRAY 1[0]":cluster{i32, "mapaeeprom":string, "mapaeeprom":string, dbl, u8, "unsigned byte array[0]":u8}}
  T26 = cluster{"Señales Logicas:[0]":cluster{i32, "mapaeeprom":string, bool}}
  T27 = cluster{"[0]":dbl, "[1]":dbl, "[2]":dbl, "[3]":dbl, "[4]":dbl, "[5]":dbl, "[6]":dbl, "[7]":dbl, "[8]":dbl}
  T28 = cluster{i32, "trimmed string":string, "trimmed string":string, dbl, u8, "unsigned byte array[0]":u8}
  T29 = cluster{i32, "trimmed string":string, "trimmed string":string, dbl, u8, "unsigned byte array[0]":u8}[]
  T30 = cluster{i32, "trimmed string":string, "trimmed string":string, dbl, u8, "unsigned byte array[0]":u8}[][]
  T31 = cluster{"mapaeeprom":string, "cantmedic":u8, "Med_nom":string[], "Med_unid":string[], "Med_caract":string}
  T32 = cluster{string, "cantmedic":u8, "Med_nom":string[], "Med_unid":string[], "Med_caract":string}
  T33 = cluster{i32, "mapaeeprom":string, "mapaeeprom":string, i32, i32, i32}
  T34 = cluster{i32, "mapaeeprom":string, "mapaeeprom":string, i32, i32, i32}[]
  T35 = cluster{"IP":string, "Puerto:":u16, "Time Out":u16}
  T36 = cluster{"Nº":i32, "Nombre":string, "Unidad":string, u8, "unsigned byte array[0]":u8, u8}[]
  T37 = cluster{i32, "mapaeeprom":string, "mapaeeprom":string, u8, "unsigned byte array[0]":u8, u8}[]
  T38 = cluster{"Rotulo 1":string, "Rotulo 2":string, "Cant. Meds.":u8, "Med ampl":u8, "Analogicas 16":cluster{i32, "mapaeeprom":string, "mapaeeprom":string, u8, "unsigned byte array[0]":u8, u8}[], "Analogicas 32":cluster{i32, "mapaeeprom":string, "mapaeeprom":string, u8, "unsigned byte array[0]":u8, u8}[], "DIG_CARACT":cluster{"ESTADO":bool, "VAL_INI":bool, "VAL_FIJO":bool, "VAL_CORTE":bool, "CARACT LOG 9-16":string}[], "DIG_CARACT 2":cluster{"ESTADO":bool, "VAL_INI":bool, "VAL_FIJO":bool, "VAL_CORTE":bool, "CARACT LOG 9-16":string}[], "PWM":cluster{"CONF_PWM1":u8, "VALOR_PWM1":u8, "CONF_PWM2":u8, "VALOR_PWM2":u8}}
  T39 = cluster{"Nº":i32, "Nombre":string, "Unidad":string, "Linealidad":dbl, "Escala":u8, "Promediacion":u8}[]
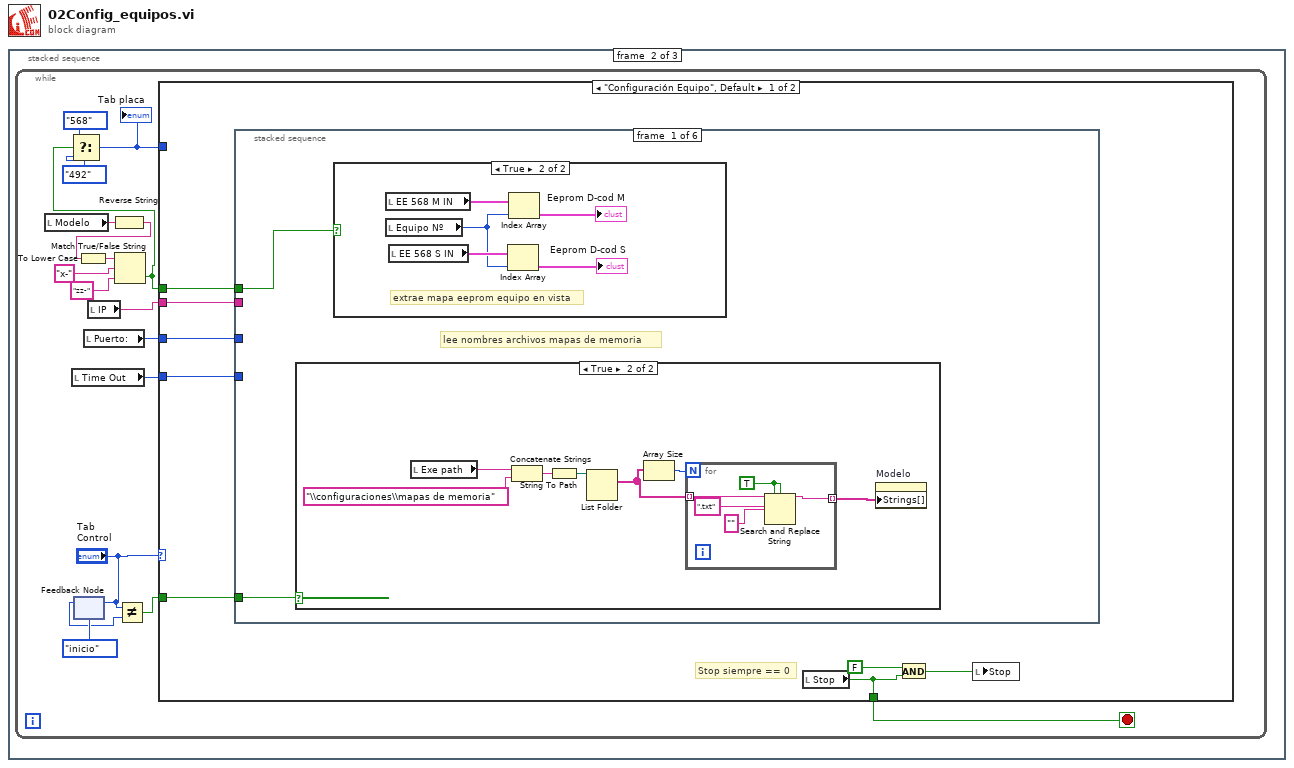
[diagram p0: block diagram]
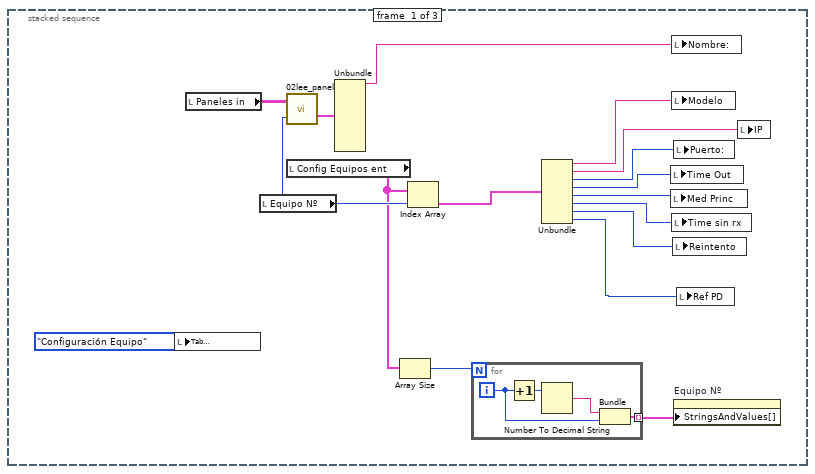
[diagram p2: hidden frame]
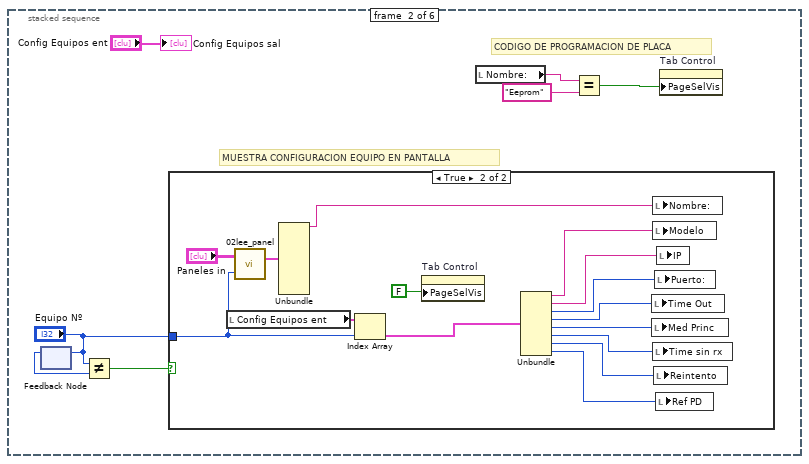
[diagram p5: hidden frame]
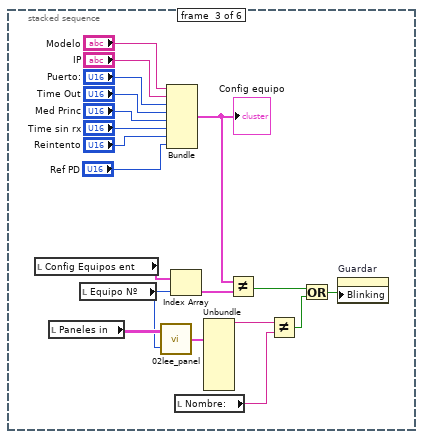
[diagram p7: hidden frame]
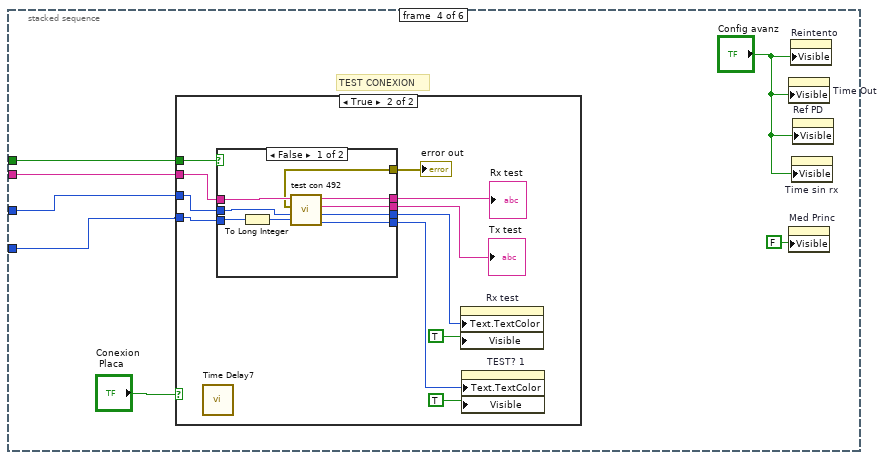
[diagram p8: hidden frame]
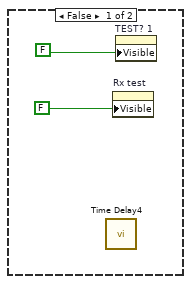
[diagram p9: hidden frame]
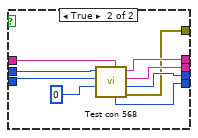
[diagram p10: hidden frame]
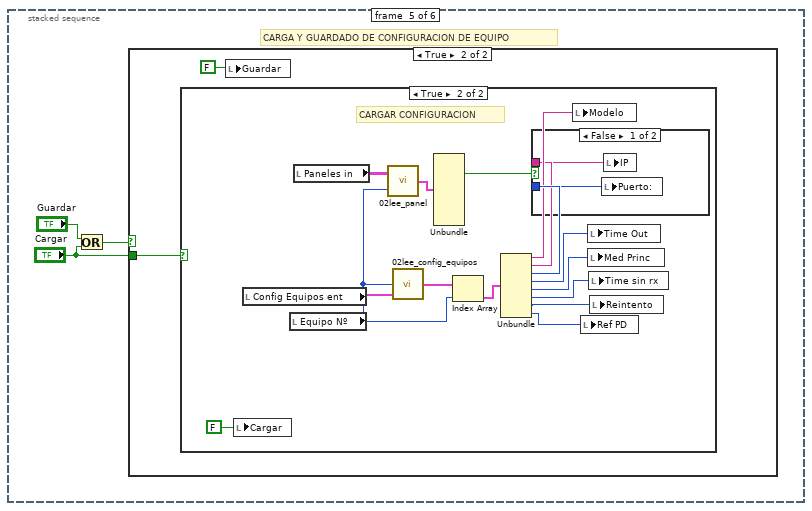
[diagram p11: hidden frame]
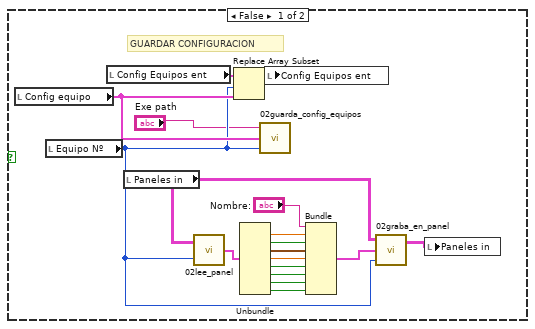
[diagram p13: hidden frame]
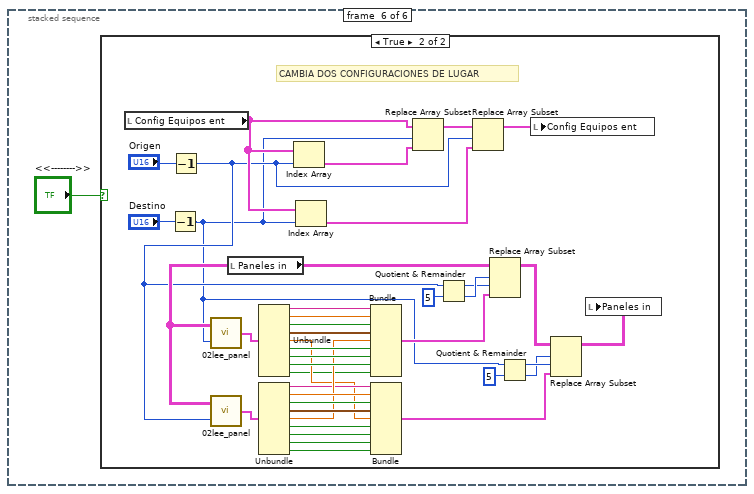
[diagram p15: hidden frame]
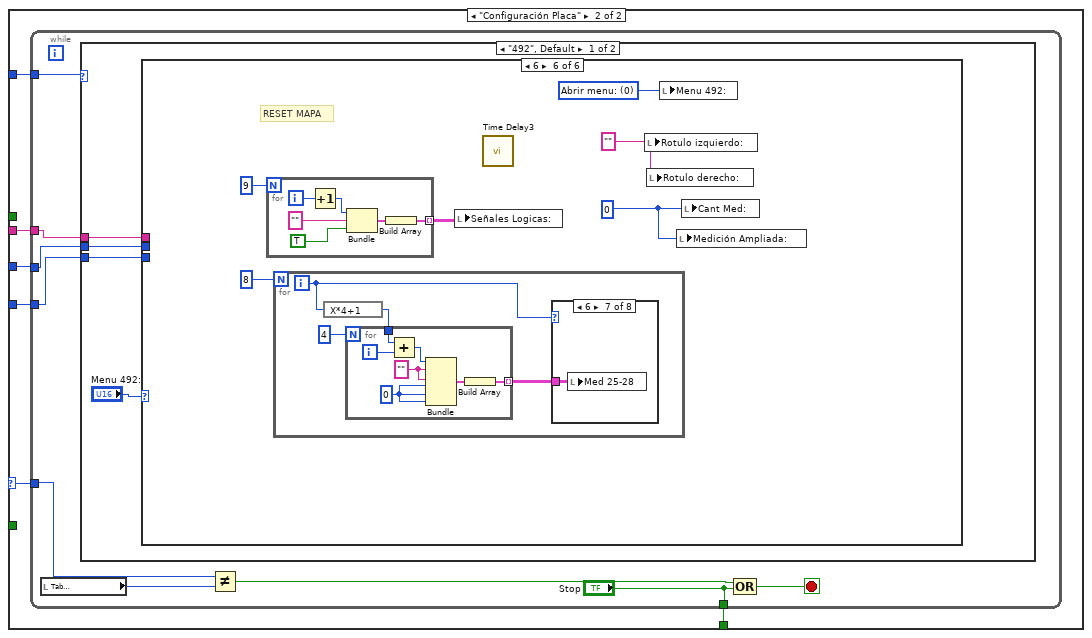
[diagram p17: hidden frame]
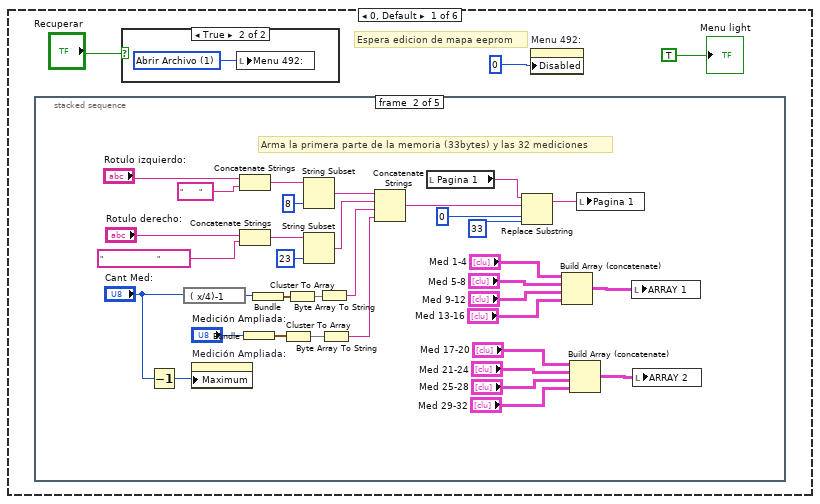
[diagram p18: hidden frame]
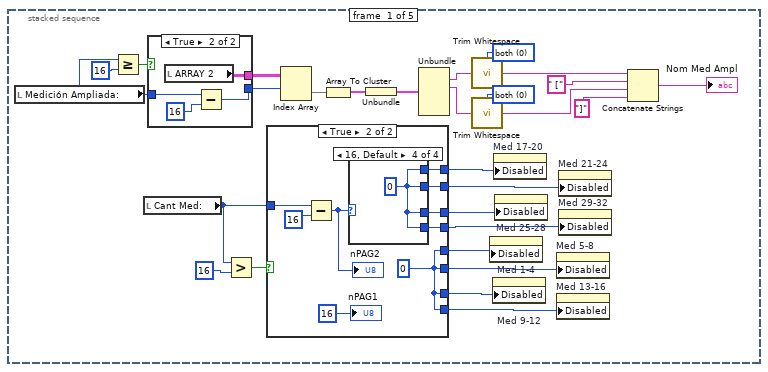
[diagram p20: hidden frame]
diagram:
  n1 = stacked-sequence {
    frame #0 {
      n2 = local write "Tab\nControl"(T9."Configuración Equipo" ("Tab\nControl")) -> ()
      n3 = local read "Paneles in"() -> (w14:T4)
      n4 = local read "Equipo Nº"() -> (w17:i32)
      n5 = call "02lee_panel.vi"("Equipo Nº"=w17, "Paneles"=w14) -> ("Panel"=w15:T16)
      n6 = local read "Config Equipos ent"() -> (w6:T6)
      n7 = Unbundle(w15) -> ("Nombre"=w13:string)  [unwired: 8 out]
      n8 = Array Size(array=w6) -> (size(s)=w3:i32)
      n9 = Index Array(array=w6, index=w17) -> (element=w16:T17)
      n10 = for {
        N: w3 -> [_]
        tunnel: [w21] -> w7 mode=indexing
        i -> [w20]
        n11 = Increment(x=w20) -> (x+1=w19:i32)
        n12 = Number To Decimal String(number=w19) -> (decimal integer string=w18:string)  [unwired: 1 out]
        n13 = Bundle(w18, w20) -> (w21:cluster{string, i32})  [unwired: 1 out]
      }
      n14 = Unbundle(w16) -> ("Modelo"=w12:string, "IP"=w11:string, "Puerto"=w10:u16, "Time Out"=w9:u16, "Med Princ"=w8:u16, "Time sin rx"=w5:u16, "Reintento"=w4:u16, "Ref PD 2"=w2:u16)
      n15 = local write "Time Out"(w9) -> ()
      n16 = local write "Med Princ"(w8) -> ()
      n17 = local write "Nombre:"(w13) -> ()
      n18 = local write "Modelo"(w12) -> ()
      n19 = local write "Time sin rx"(w5) -> ()
      n20 = local write "Reintento"(w4) -> ()
      n21 = local write "Puerto:"(w10) -> ()
      n22 = property on="Equipo Nº" class="Ring (strict)"("StringsAndValues[]"=w7) -> ()  [unwired: 2 in, 2 out]
      n23 = local write "Ref PD"(w2) -> ()
      n24 = local write "IP"(w11) -> ()
    }
    frame #1 {
      n25 = while {
        stop <- w38 stop-if-true
        n26 = local read "Modelo"() -> (w29:string)
        n27 = local read "Time Out"() -> (w37:u16)
        n28 = feedback #1(T14."inicio" ("Tab\n Control")) -> (w33:T14)
        n29 = feedback-in #1("Tab\nControl") -> ()
        n30 = local read "Puerto:"() -> (w36:u16)
        n31 = local read "IP"() -> (w35:string)
        n32 = Reverse String(1:w29) -> (0:w28:string)
        n33 = To Lower Case(string=w28) -> (all lower case string=w27:string)
        n34 = Match True/False String(2:"zz-" ("y"), 3:"x-" ("y"), 4:w27) -> (0:w25:bool)  [unwired: 1 out]
        n35 = Select(t=enum32{"492", "568"}."568" ("Tab placa"), s=w25, f=enum32{"492", "568"}."492" ("Tab placa")) -> (s? t:f=w22:enum32{"492", "568"})
        "Tab placa" <- w22
        n36 = Not Equal?(x="Tab\nControl", y=w33) -> (x != y?=w31:bool)
        n37 = case shown="\"Configuración Equipo\", Default" "Tab\nControl" {
          selector: "Tab\nControl" -> [_ w231]
          tunnel: [w42 w232] -> w38
          tunnel: w35 -> [w46 w230]
          tunnel: w37 -> [w45 w229]
          tunnel: w36 -> [w44 w228]
          tunnel: w31 -> [w40 _]
          tunnel: w25 -> [w39 _]
          tunnel: w22 -> [_ w227]
          frame "Configuración Equipo", Default {
            # "Stop siempre == 0"
            n38 = stacked-sequence {
              tunnel: w46 -> [_ _ _ w112 _ _]
              tunnel: w44 -> [_ _ _ w111 _ _]
              tunnel: w45 -> [_ _ _ w108 _ _]
              tunnel: w40 -> [w48 _ _ _ _ _]
              tunnel: w39 -> [w47 _ _ w107 _ _]
              frame #0 {
                # "lee nombres archivos mapas de memoria"
                n39 = case shown="True" w48 {
                  frame False {
                  }
                  frame True {
                    n40 = local read "Exe path"() -> (w57:string)
                    n41 = Concatenate Strings(w57, "\\configuraciones\\mapas de memoria") -> (w59:string)
                    n42 = String To Path(string=w59) -> (path=w60:path)
                    n43 = List Folder(path=w60) -> (filenames=w55:string[])  [unwired: 3 in, 3 out]
                    n44 = Array Size(array=w55) -> (size(s)=w56:i32)
                    n45 = for {
                      N: w56 -> [_]
                      tunnel: w55 -> [w65] mode=indexing
                      tunnel: [w62] -> w54 mode=indexing
                      w61 = TRUE ("replace all? (F)")
                      n46 = Search and Replace String(replace all?=w61, case sensitive?=w61, input string=w65, search string=".txt", replace string="" ("replace string (\"\")")) -> (result string=w62:string)  [unwired: 3 in, 3 out]
                    }
                    n47 = property on="Modelo" class="CmbBox"("Strings[]"=w54) -> ()  [unwired: 2 in, 2 out]
                  }
                }
                n48 = case shown="True" w47 {
                  frame False {
                  }
                  frame True {
                    # "extrae mapa eeprom equipo en vista"
                    n49 = local read "EE 568 M IN"() -> (w53:T2)
                    n50 = local read "Equipo Nº"() -> (w51:i32)
                    n51 = local read "EE 568 S IN"() -> (w52:T2)
                    n52 = Index Array(array=w52, index=w51) -> (element=→"Eeprom D-cod S":T1)
                    n53 = Index Array(array=w53, index=w51) -> (element=→"Eeprom D-cod M":T1)
                  }
                }
              }
              frame #1 {
                # "CODIGO DE PROGRAMACION DE PLACA"
                # "MUESTRA CONFIGURACION EQUIPO EN PANTALLA"
                n54 = feedback-in #2("Equipo Nº") -> ()
                n55 = feedback #2() -> (w72:i32)  [unwired: 1 out]
                n56 = Not Equal?(x="Equipo Nº", y=w72) -> (x != y?=w70:bool)
                n57 = case shown="True" w70 {
                  tunnel: "Equipo Nº" -> [_ w85]
                  frame False {
                  }
                  frame True {
                    n58 = local read "Config Equipos ent"() -> (w86:T6)
                    n59 = call "02lee_panel.vi"("Equipo Nº"=w85, "Paneles"="Paneles in") -> ("Panel"=w84:T16)
                    n60 = Unbundle(w84) -> ("Nombre"=w83:string)  [unwired: 8 out]
                    n61 = Index Array(array=w86, index=w85) -> (element=w87:T17)
                    n62 = property on="Tab Control" class="TabCtl (strict)"("PageSelVis"=FALSE) -> ()  [unwired: 2 in, 2 out]
                    n63 = Unbundle(w87) -> ("Modelo"=w82:string, "IP"=w81:string, "Puerto"=w80:u16, "Time Out"=w79:u16, "Med Princ"=w78:u16, "Time sin rx"=w76:u16, "Reintento"=w75:u16, "Ref PD 2"=w74:u16)
                    n64 = local write "Time Out"(w79) -> ()
                    n65 = local write "Med Princ"(w78) -> ()
                    n66 = local write "Nombre:"(w83) -> ()
                    n67 = local write "Modelo"(w82) -> ()
                    n68 = local write "Time sin rx"(w76) -> ()
                    n69 = local write "Reintento"(w75) -> ()
                    n70 = local write "Puerto:"(w80) -> ()
                    n71 = local write "Ref PD"(w74) -> ()
                    n72 = local write "IP"(w81) -> ()
                  }
                }
                n73 = local read "Nombre:"() -> (w68:string)
                n74 = Equal?(x=w68, y="Eeprom") -> (x = y?=w67:bool)
                n75 = property on="Tab Control" class="TabCtl (strict)"("PageSelVis"=w67) -> ()  [unwired: 2 in, 2 out]
                "Config Equipos sal" <- "Config Equipos ent"
              }
              frame #2 {
                n76 = local read "Config Equipos ent"() -> (w100:T6)
                n77 = local read "Paneles in"() -> (w95:T4)
                n78 = local read "Equipo Nº"() -> (w94:i32)
                n79 = call "02lee_panel.vi"("Equipo Nº"=w94, "Paneles"=w95) -> ("Panel"=w93:T16)
                n80 = Bundle("Modelo"="Modelo", "IP"="IP", "Puerto:"="Puerto:", "Time Out"="Time Out", "Med Princ"="Med Princ", "Time sin rx"="Time sin rx", "Reintento"="Reintento", "Ref PD"="Ref PD") -> (w101:T18)  [unwired: 1 out]
                "Config equipo" <- w101
                n81 = Index Array(array=w100, index=w94) -> (element=w99:T17)
                n82 = local read "Nombre:"() -> (w91:string)
                n83 = Unbundle(w93) -> ("Nombre"=w92:string)  [unwired: 8 out]
                n84 = Not Equal?(x=w101, y=w99) -> (x != y?=w98:bool)
                n85 = Not Equal?(x=w92, y=w91) -> (x != y?=w97:bool)
                n86 = Or(x=w98, y=w97) -> (x .or. y?=w96:bool)
                n87 = property on="Guardar" class="Bool (strict)"("Blinking"=w96) -> ()  [unwired: 2 in, 2 out]
              }
              frame #3 {
                # "TEST CONEXION"
                n88 = case shown="True" "Conexion\n Placa" {
                  tunnel: w112 -> [_ w126]
                  tunnel: w111 -> [_ w125]
                  tunnel: w108 -> [_ w120]
                  tunnel: w107 -> [_ w116]
                  frame False {
                    n89 = call "Time Delay4"() -> ()  [unwired: 2 in, 10 out]
                    n90 = property on="Rx test" class="Str"("Visible"=FALSE) -> ()  [unwired: 2 in, 2 out]
                    n91 = property on="TEST? 1" class="Str"("Visible"=FALSE) -> ()  [unwired: 2 in, 2 out]
                  }
                  frame True {
                    n92 = call "Time Delay7"() -> ()  [unwired: 2 in, 10 out]
                    n93 = case shown="False" w116 {
                      tunnel: w126 -> [w135 w142]
                      tunnel: w125 -> [w134 w144]
                      tunnel: [w133 w139] -> w119
                      tunnel: [w132 w138] -> w118
                      tunnel: [w131 w140] -> w123
                      tunnel: [w130 w141] -> w122
                      tunnel: w120 -> [w129 w143]
                      tunnel: [w127 w136] -> w117
                      frame False {
                        n94 = To Long Integer(number=w129) -> (32bit integer=w128:i32)
                        n95 = call "test con 492.vi"("Numeric"=w128, "Puerto:"=w134, "IP"=w135) -> ("Text.Text Colors:Text Color"=w132:u32, "Text.Text Colors:Text Color 2"=w133:u32, "TEST? 2"=w131:string, "TEST?"=w130:string, "error out"=w127:errorcluster)
                      }
                      frame True {
                        n96 = call "Test con 568.vi"("Equipo Nº"=u8 0, "Time Out"=w143, "Puerto:"=w144, "IP"=w142) -> ("Tx test color"=w138:u32, "error out"=w136:errorcluster, "RX tets color"=w139:u32, "SEND"=w140:string, "RETURN"=w141:string)  [unwired: 1 in]
                      }
                    }
                    "Rx test" <- w122
                    "Tx test" <- w123
                    "error out" <- w117
                    n97 = property on="Rx test" class="Str"("Text.TextColor"=w119, "Visible"=TRUE) -> ()  [unwired: 2 in, 2 out]
                    n98 = property on="TEST? 1" class="Str"("Text.TextColor"=w118, "Visible"=TRUE) -> ()  [unwired: 2 in, 2 out]
                  }
                }
                n99 = property on="Time Out" class="DigNum (strict)"("Visible"="Config avanz") -> ()  [unwired: 2 in, 2 out]
                n100 = property on="Med Princ" class="Ring (strict)"("Visible"=FALSE) -> ()  [unwired: 2 in, 2 out]
                n101 = property on="Reintento" class="DigNum (strict)"("Visible"="Config avanz") -> ()  [unwired: 2 in, 2 out]
                n102 = property on="Time sin rx" class="DigNum (strict)"("Visible"="Config avanz") -> ()  [unwired: 2 in, 2 out]
                n103 = property on="Ref PD" class="DigNum (strict)"("Visible"="Config avanz") -> ()  [unwired: 2 in, 2 out]
              }
              frame #4 {
                # "CARGA Y GUARDADO DE CONFIGURACION DE EQUIPO"
                n104 = Or(x="Guardar", y="Cargar") -> (x .or. y?=w146:bool)
                n105 = case shown="True" w146 {
                  tunnel: "Cargar" -> [_ w149]
                  frame False {
                  }
                  frame True {
                    n106 = case shown="True" w149 {
                      frame False {
                        # "GUARDAR CONFIGURACION"
                        n107 = local read "Config equipo"() -> (w165:T7)
                        n108 = local read "Equipo Nº"() -> (w156:i32)
                        n109 = local read "Config Equipos ent"() -> (w167:T6)
                        n110 = local read "Paneles in"() -> (w164:T4)
                        n111 = call "02lee_panel.vi"("Equipo Nº"=w156, "Paneles"=w164) -> ("Panel"=w163:T16)
                        n112 = Replace Array Subset(array=w167, new element=w165, index=w156) -> (w166:T6)
                        n113 = Unbundle(w163) -> ("Med\nprinc"=w159:dbl, "On/Off"=w160:bool, "Ultima recepción"=w161:timestamp, "Nº"=w162:dbl, "deshabilitacion"=w154:bool, "Actividad"=w153:bool, "falla"=w152:bool, "alarm"=w150:bool)  [unwired: 1 out]
                        n114 = call "02guarda_config_equipos.vi"("Nº equipo"=w156, "Config equipo"=w165, "exe path"="Exe path") -> ()  [unwired: 1 out]
                        n115 = local write "Config Equipos ent"(w166) -> ()
                        n116 = Bundle("Nombre:"="Nombre:", "Med\nprinc"=w159, "On/Off"=w160, "Ultima recepción"=w161, "Nº"=w162, "deshabilitacion"=w154, "Actividad"=w153, "falla"=w152, "alarm"=w150) -> (w157:T19)  [unwired: 1 out]
                        n117 = call "02graba_en_panel.vi"("Equipo Nº"=w156, "Panel"=w157, "Paneles in"=w164) -> ("Paneles out"=w155:T20)  [unwired: 1 out]
                        n118 = local write "Paneles in"(w155) -> ()
                      }
                      frame True {
                        # "CARGAR CONFIGURACION"
                        n119 = local write "Cargar"(FALSE ("Cargar")) -> ()
                        n120 = local read "Config Equipos ent"() -> (w172:T6)
                        n121 = local read "Equipo Nº"() -> (w171:i32)
                        n122 = local read "Paneles in"() -> (w176:T4)
                        n123 = call "02lee_panel.vi"("Equipo Nº"=w171, "Paneles"=w176) -> ("Panel"=w175:T16)
                        n124 = call "02lee_config_equipos.vi"("Config Equipos ent"=w172, "Equipo Nº"=w171) -> ("Config Equipos sal"=w173:T6)  [unwired: 1 in]
                        n125 = Unbundle(w175) -> ("On/Off"=w174:bool)  [unwired: 8 out]
                        n126 = Index Array(array=w173, index=w171) -> (element=w182:T17)
                        n127 = Unbundle(w182) -> ("Modelo"=w178:string, "IP"=w177:string, "Puerto"=w179:u16, "Time Out"=w180:u16, "Med Princ"=w181:u16, "Time sin rx"=w170:u16, "Reintento"=w169:u16, "Ref PD 2"=w168:u16)
                        n128 = case shown="False" w174 {
                          tunnel: w179 -> [w185 _]
                          tunnel: w177 -> [w184 _]
                          frame False {
                            n129 = local write "Puerto:"(w185) -> ()
                            n130 = local write "IP"(w184) -> ()
                          }
                          frame True {
                          }
                        }
                        n131 = local write "Modelo"(w178) -> ()
                        n132 = local write "Ref PD"(w168) -> ()
                        n133 = local write "Time Out"(w180) -> ()
                        n134 = local write "Med Princ"(w181) -> ()
                        n135 = local write "Time sin rx"(w170) -> ()
                        n136 = local write "Reintento"(w169) -> ()
                      }
                    }
                    n137 = local write "Guardar"(FALSE ("Cargar")) -> ()
                  }
                }
              }
              frame #5 {
                n138 = case shown="True" "<<-------->>" {
                  frame False {
                  }
                  frame True {
                    # "CAMBIA DOS CONFIGURACIONES DE LUGAR"
                    n139 = local read "Config Equipos ent"() -> (w226:T6)
                    n140 = Decrement(x="Destino") -> (x-1=w190:u16)
                    n141 = Decrement(x="Origen") -> (x-1=w191:u16)
                    n142 = local read "Paneles in"() -> (w199:T4)
                    n143 = call "02lee_panel.vi"("Equipo Nº"=w190, "Paneles"=w199) -> ("Panel"=w221:T16)
                    n144 = call "02lee_panel.vi"("Equipo Nº"=w191, "Paneles"=w199) -> ("Panel"=w208:T16)
                    n145 = Unbundle(w221) -> ("Nombre"=w195:string, "Med\nprinc"=w218:dbl, "On/Off"=w219:bool, "Ultima recepción"=w220:timestamp, "Nº"=w193:dbl, "deshabilitacion"=w217:bool, "Actividad"=w216:bool, "falla"=w215:bool, "alarm"=w187:bool)
                    n146 = Unbundle(w208) -> ("Nombre"=w194:string, "Med\nprinc"=w211:dbl, "On/Off"=w210:bool, "Ultima recepción"=w209:timestamp, "Nº"=w196:dbl, "deshabilitacion"=w212:bool, "Actividad"=w213:bool, "falla"=w214:bool, "alarm"=w188:bool)
                    n147 = Index Array(array=w226, index=w191) -> (element=w225:T17)
                    n148 = Index Array(array=w226, index=w190) -> (element=w223:T17)
                    n149 = Bundle("Nombre"=w195, "Med\nprinc"=w218, "On/Off"=w219, "Ultima recepción"=w220, "Nº"=w196, "deshabilitacion"=w217, "Actividad"=w216, "falla"=w215, "alarm"=w187) -> (w198:T16)  [unwired: 1 out]
                    n150 = Bundle("Nombre"=w194, "Med\nprinc"=w211, "On/Off"=w210, "Ultima recepción"=w209, "Nº"=w193, "deshabilitacion"=w212, "Actividad"=w213, "falla"=w214, "alarm"=w188) -> (w197:T16)  [unwired: 1 out]
                    n151 = Replace Array Subset(array=w226, new element=w225, index=w190) -> (w224:T6)
                    n152 = Quotient & Remainder(x=w191, y=5) -> (x-y*floor(x/y)=w205:i32, floor(x/y)=w206:i32)
                    n153 = Replace Array Subset(array=w224, new element=w223, index=w191) -> (w222:T6)
                    n154 = Replace Array Subset(array=w199, new element=w198, index (row)=w206, index (col)=w205) -> (w201:T4)
                    n155 = Quotient & Remainder(x=w190, y=5) -> (x-y*floor(x/y)=w204:i32, floor(x/y)=w203:i32)
                    n156 = local write "Config Equipos ent"(w222) -> ()
                    n157 = Replace Array Subset(array=w201, new element=w197, index (row)=w203, index (col)=w204) -> (w200:T4)
                    n158 = local write "Paneles in"(w200) -> ()
                  }
                }
              }
            }
            n159 = local read "Stop"() -> (w42:bool)
            n160 = And(x=FALSE, y=w42) -> (x .and. y?=w43:bool)
            n161 = local write "Stop"(w43) -> ()
          }
          frame "Configuración Placa" {
            n162 = while {
              tunnel: ["Stop"] -> w232
              tunnel: w231 -> [w239]
              tunnel: w228 -> [w236]
              tunnel: w230 -> [w235]
              tunnel: w229 -> [w234]
              tunnel: w227 -> [w233]
              stop <- w241 stop-if-true
              n163 = local read "Tab\nControl"() -> (w240:T9)
              n164 = case shown="\"492\", Default" w233 {
                tunnel: w236 -> [w245 w803]
                tunnel: w235 -> [w244 w804]
                tunnel: w234 -> [w243 w802]
                frame "492", Default {
                  n165 = case shown="6" "Menu 492:" {
                    selector: "Menu 492:" -> [_ w503 _ _ _ _]
                    tunnel: w245 -> [_ w501 _ w747 _ _]
                    tunnel: w244 -> [_ w502 _ w746 _ _]
                    tunnel: w243 -> [_ w500 _ w748 _ _]
                    frame 0, Default {
                      # "Espera edicion de mapa eeprom"
                      n166 = stacked-sequence {
                        frame #0 {
                          w277 = T21 0 items=["both", "start of string", "end of string"] ("location (both)")
                          w272 = T21 0 items=["both", "start of string", "end of string"] ("location (both)")
                          n167 = local read "Medición Ampliada:"() -> (w268:u8)
                          n168 = Greater Or Equal?(x=w268, y=u8 16) -> (x >= y?=w266:bool)
                          n169 = local read "Cant Med:"() -> (w259:u8)
                          n170 = case shown="True" w266 {
                            tunnel: [w310 w314] -> w265
                            tunnel: [w309 w313] -> w261
                            tunnel: w268 -> [w309 w312]
                            frame False {
                              n171 = local read "ARRAY 1"() -> (w310:T8)
                            }
                            frame True {
                              n172 = local read "ARRAY 2"() -> (w314:T8)
                              n173 = Subtract(x=w312, y=u8 16) -> (x-y=w313:u8)
                            }
                          }
                          n174 = Greater?(x=w259, y=u8 16) -> (0:w251:bool)
                          n175 = case shown="True" w251 {
                            tunnel: w259 -> [w278 w293]
                            tunnel: [w283 w299] -> w258
                            tunnel: [w283 w298] -> w257
                            tunnel: [w283 w297] -> w256
                            tunnel: [w283 w296] -> w255
                            tunnel: [w279 w300] -> w252
                            tunnel: [w282 w300] -> w260
                            tunnel: [w281 w300] -> w253
                            tunnel: [w280 w300] -> w254
                            frame False {
                              w283 = u8 2 ("PAG2")
                              n176 = local write "nPAG1"(w278) -> ()
                              n177 = case shown="4" w278 {
                                tunnel: [w285 u8 0 ("PAG2") w289 w291 w292] -> w279
                                tunnel: [w285 w286 w289 w291 w292] -> w282
                                tunnel: [w285 w286 w288 w291 w292] -> w281
                                tunnel: [w285 w286 w288 u8 2 ("PAG2") w292] -> w280
                                frame 0 {
                                w285 = u8 2 ("PAG2")
                                }
                                frame 4 {
                                w286 = u8 2 ("PAG2")
                                }
                                frame 8 {
                                w289 = u8 0 ("PAG2")
                                w288 = u8 2 ("PAG2")
                                }
                                frame 12 {
                                w291 = u8 0 ("PAG2")
                                }
                                frame 16, Default {
                                w292 = u8 0 ("PAG2")
                                }
                              }
                              n178 = local write "nPAG2"(u8 0 ("PAG2")) -> ()
                            }
                            frame True {
                              w300 = u8 0 ("PAG1")
                              n179 = Subtract(x=w293, y=u8 16) -> (x-y=w294:u8)
                              "nPAG2" <- w294
                              n180 = case shown="16, Default" w294 {
                                tunnel: [u8 0 ("PAG2") w305 w307 w308] -> w299
                                tunnel: [w302 w305 w307 w308] -> w298
                                tunnel: [w302 w304 w307 w308] -> w297
                                tunnel: [w302 w304 u8 2 ("PAG2") w308] -> w296
                                frame 4 {
                                w302 = u8 2 ("PAG2")
                                }
                                frame 8 {
                                w305 = u8 0 ("PAG2")
                                w304 = u8 2 ("PAG2")
                                }
                                frame 12 {
                                w307 = u8 0 ("PAG2")
                                }
                                frame 16, Default {
                                w308 = u8 0 ("PAG2")
                                }
                              }
                              "nPAG1" <- u8 16 ("PAG1")
                            }
                          }
                          n181 = Index Array(array=w265, index (row)=w261) -> (element=w264:T22)  [unwired: 1 in]
                          n182 = Array To Cluster(array=w264) -> (cluster=w263:T23)
                          n183 = Unbundle(w263) -> ("ARRAY 2[0]"=w262:T24)
                          n184 = Unbundle(w262) -> ("mapaeeprom"=w275:string, "mapaeeprom"=w271:string)  [unwired: 4 out]
                          n185 = call <vilib>:"Trim Whitespace.vi"("string"=w275, "location (both)"=w277) -> ("trimmed string"=w276:string)
                          n186 = call <vilib>:"Trim Whitespace.vi"("string"=w271, "location (both)"=w272) -> ("trimmed string"=w273:string)
                          n187 = property on="Med 1-4" class="Arr (strict)"("Disabled"=w252) -> ()  [unwired: 2 in, 2 out]
                          n188 = property on="Med 9-12" class="Arr (strict)"("Disabled"=w253) -> ()  [unwired: 2 in, 2 out]
                          n189 = property on="Med 17-20" class="Arr (strict)"("Disabled"=w258) -> ()  [unwired: 2 in, 2 out]
                          n190 = property on="Med 25-28" class="Arr (strict)"("Disabled"=w256) -> ()  [unwired: 2 in, 2 out]
                          n191 = property on="Med 5-8" class="Arr (strict)"("Disabled"=w260) -> ()  [unwired: 2 in, 2 out]
                          n192 = property on="Med 13-16" class="Arr (strict)"("Disabled"=w254) -> ()  [unwired: 2 in, 2 out]
                          n193 = property on="Med 21-24" class="Arr (strict)"("Disabled"=w257) -> ()  [unwired: 2 in, 2 out]
                          n194 = property on="Med 29-32" class="Arr (strict)"("Disabled"=w255) -> ()  [unwired: 2 in, 2 out]
                          n195 = Concatenate Strings(w276, " [" ("string"), w273, "]" ("string")) -> (→"Nom Med Ampl":string)
                        }
                        frame #1 {
                          # "Arma la primera parte de la memoria (33bytes) y las 32 mediciones"
                          n196 = Decrement(x="Cant Med:") -> (x-1=w315:u8)
                          n197 = expression code="( x/4)-1"("Cant Med:") -> (w349:u8)
                          n198 = property on="Medición Ampliada:" class="Ring (strict)"("Maximum"=w315) -> ()  [unwired: 2 in, 2 out]
                          n199 = Concatenate Strings("Rotulo izquierdo:", "        " ("string")) -> (w340:string)
                          n200 = Concatenate Strings("Rotulo derecho:", "                           " ("string")) -> (w339:string)
                          n201 = Bundle("Medición Ampliada:"="Medición Ampliada:") -> (w345:cluster{"Medición Ampliada:":u8})  [unwired: 1 in]
                          n202 = Bundle("Cant Med:"=w349) -> (w347:cluster{"Cant Med:":u8})  [unwired: 1 in]
                          n203 = Cluster To Array(cluster=w345) -> (array=w344:u8[])
                          n204 = Cluster To Array(cluster=w347) -> (array=w346:u8[])
                          n205 = String Subset(string=w340, length (rest)=8 ("length (rest)")) -> (substring=w335:string)  [unwired: 1 out]
                          n206 = String Subset(string=w339, length (rest)=23 ("length (rest)")) -> (substring=w336:string)  [unwired: 1 out]
                          n207 = Byte Array To String(unsigned byte array=w346) -> (string=w348:string)
                          n208 = Byte Array To String(unsigned byte array=w344) -> (string=w343:string)
                          n209 = Concatenate Strings(w335, w336, w348, w343) -> (w333:string)
                          n210 = local read "Pagina 1"() -> (w334:string)
                          n211 = Replace Substring(2:33 ("length (len. of substring)"), 3:0 ("offset (0)"), 4:w333, 5:w334) -> (1:w330:string)  [unwired: 1 out]
                          n212 = Build Array (concatenate)("Med 1-4", "Med 5-8", "Med 9-12", "Med 13-16") -> (w329:T10)
                          n213 = Build Array (concatenate)("Med 17-20", "Med 21-24", "Med 25-28", "Med 29-32") -> (w328:T10)
                          n214 = local write "Pagina 1"(w330) -> ()
                          n215 = local write "ARRAY 1"(w329) -> ()
                          n216 = local write "ARRAY 2"(w328) -> ()
                        }
                        frame #2 {
                          n217 = local read "nPAG1"() -> (w351:u8)
                          n218 = local read "nPAG2"() -> (w350:u8)
                          n219 = for {
                            N: w351 -> [_]
                            i -> [w391]
                            n220 = Index Array(array="ARRAY 1", index (row)=w391) -> (element=w419:T22)  [unwired: 1 in]
                            n221 = Array To Cluster(array=w419) -> (cluster=w418:T25)
                            n222 = Unbundle(w418) -> ("ARRAY 1[0]"=w410:T24)
                            n223 = Unbundle(w410) -> ("mapaeeprom"=w388:string, "mapaeeprom"=w387:string, w397:dbl, w398:u8, "unsigned byte array[0]"=w399:u8)  [unwired: 1 out]
                            n224 = Multiply(x=w397, y=u16 16) -> (x*y=w406:dbl)
                            n225 = Add(x=w406, y=w398) -> (x+y=w405:dbl)
                            n226 = Bundle(w405) -> (w404:cluster{dbl})  [unwired: 1 in]
                            n227 = Bundle("unsigned byte array[0]"=w399) -> (w400:cluster{"unsigned byte array[0]":u8})  [unwired: 1 in]
                            n228 = Concatenate Strings(w388, "       " ("string")) -> (w415:string)
                            n229 = Concatenate Strings(w387, "   " ("string")) -> (w412:string)
                            n230 = Cluster To Array(cluster=w404) -> (array=w403:dbl[])
                            n231 = Cluster To Array(cluster=w400) -> (array=w401:u8[])
                            n232 = String Subset(string=w412, length (rest)=3 ("length (rest)")) -> (substring=w409:string)  [unwired: 1 out]
                            n233 = String Subset(string=w415, length (rest)=7 ("length (rest)")) -> (substring=w408:string)  [unwired: 1 out]
                            n234 = Byte Array To String(unsigned byte array=w403) -> (string=w402:string)
                            n235 = Byte Array To String(unsigned byte array=w401) -> (string=w396:string)
                            n236 = Concatenate Strings(w408, w409, w402, w396) -> (w417:string)
                            n237 = expression code="33+(x*12)"(w391) -> (w390:i32)
                            n238 = local read "Pagina 1"() -> (w395:string)
                            n239 = String Subset(string=w417, offset (0)=0, length (rest)=12 ("length (rest)")) -> (substring=w394:string)
                            n240 = Replace Substring(2:12 ("length (len. of substring)"), 3:w390, 4:w394, 5:w395) -> (1:w393:string)  [unwired: 1 out]
                            n241 = local write "Pagina 1"(w393) -> ()
                          }
                          n242 = for {
                            N: w350 -> [_]
                            i -> [w355]
                            n243 = Index Array(array="ARRAY 2", index (row)=w355) -> (element=w384:T22)  [unwired: 1 in]
                            n244 = Array To Cluster(array=w384) -> (cluster=w383:T23)
                            n245 = Unbundle(w383) -> ("ARRAY 2[0]"=w375:T24)
                            n246 = Unbundle(w375) -> ("mapaeeprom"=w353:string, "mapaeeprom"=w352:string, w362:dbl, w363:u8, "unsigned byte array[0]"=w364:u8)  [unwired: 1 out]
                            n247 = Multiply(x=w362, y=u16 16) -> (x*y=w371:dbl)
                            n248 = Add(x=w371, y=w363) -> (x+y=w370:dbl)
                            n249 = Bundle("unsigned byte array[0]"=w364) -> (w365:cluster{"unsigned byte array[0]":u8})  [unwired: 1 in]
                            n250 = Bundle(w370) -> (w369:cluster{dbl})  [unwired: 1 in]
                            n251 = Concatenate Strings(w353, "       " ("string")) -> (w380:string)
                            n252 = Concatenate Strings(w352, "   " ("string")) -> (w377:string)
                            n253 = Cluster To Array(cluster=w369) -> (array=w368:dbl[])
                            n254 = Cluster To Array(cluster=w365) -> (array=w366:u8[])
                            n255 = String Subset(string=w380, length (rest)=7 ("length (rest)")) -> (substring=w373:string)  [unwired: 1 out]
                            n256 = String Subset(string=w377, length (rest)=3 ("length (rest)")) -> (substring=w374:string)  [unwired: 1 out]
                            n257 = Byte Array To String(unsigned byte array=w368) -> (string=w367:string)
                            n258 = Byte Array To String(unsigned byte array=w366) -> (string=w361:string)
                            n259 = Concatenate Strings(w373, w374, w367, w361) -> (w382:string)
                            n260 = expression code="x*12"(w355) -> (w357:i32)
                            n261 = local read "Pagina 2"() -> (w360:string)
                            n262 = String Subset(string=w382, offset (0)=0, length (rest)=12 ("length (rest)")) -> (substring=w356:string)
                            n263 = Replace Substring(2:12 ("length (len. of substring)"), 3:w357, 4:w356, 5:w360) -> (1:w359:string)  [unwired: 1 out]
                            n264 = local write "Pagina 2"(w359) -> ()
                          }
                        }
                        frame #3 {
                          # "Variable a usar para codificar las placas"
                          # "Ultima parte de las pag1 y pag 2: Señales logicas"
                          n265 = for {
                            N: 9 ("Numeric") -> [_]
                            tunnel: [w460] -> w450 mode=indexing
                            i -> [w455]
                            n266 = Greater Or Equal?(x=w455, y=6) -> (x >= y?=w461:bool)
                            n267 = Index Array(array="Señales Logicas:", index (row)=w455) -> (element=w467:cluster{i32, "mapaeeprom":string, bool}[])  [unwired: 1 in]
                            n268 = Array To Cluster(array=w467) -> (cluster=w466:T26)
                            n269 = Unbundle(w466) -> ("Señales Logicas:[0]"=w465:cluster{i32, "mapaeeprom":string, bool})
                            n270 = Unbundle(w465) -> ("mapaeeprom"=w452:string, w463:bool)  [unwired: 1 out]
                            n271 = case shown="False" w461 {
                              tunnel: w463 -> [w473 w482]
                              tunnel: [w472 w481] -> w460
                              tunnel: w455 -> [w471 w480]
                              frame False {
                                n272 = case shown="True" w473 {
                                tunnel: w471 -> [_ w476]
                                tunnel: [0.0 w475] -> w472
                                frame False {
                                }
                                frame True {
                                n273 = Scale By Power Of 2(n=w476, x=1.0) -> (x*2^n=w475:dbl)
                                }
                                }
                              }
                              frame True {
                                n274 = Subtract(x=w480, y=6) -> (x-y=w478:i32)
                                n275 = case shown="True" w482 {
                                tunnel: w478 -> [_ w485]
                                tunnel: [0.0 w484] -> w481
                                frame False {
                                }
                                frame True {
                                n276 = Scale By Power Of 2(n=w485, x=1.0) -> (x*2^n=w484:dbl)
                                }
                                }
                              }
                            }
                            n277 = Concatenate Strings(w452, "       " ("string")) -> (w468:string)
                            n278 = expression code="192+(x*7)"(w455) -> (w454:i32)
                            n279 = local read "Pagina 2"() -> (w459:string)
                            n280 = String Subset(string=w468, offset (0)=0, length (rest)=7 ("length (rest)")) -> (substring=w458:string)
                            n281 = Replace Substring(2:7 ("length (len. of substring)"), 3:w454, 4:w458, 5:w459) -> (1:w456:string)  [unwired: 1 out]
                            n282 = local write "Pagina 2"(w456) -> ()
                          }
                          n283 = Compound Arithmetic op=ADD(w450) -> (w449:dbl[])
                          n284 = Array To Cluster(array=w449) -> (cluster=w448:T27)
                          n285 = Unbundle(w448) -> ("[0]"=w447:dbl, "[1]"=w446:dbl, "[2]"=w445:dbl, "[3]"=w444:dbl, "[4]"=w443:dbl, "[5]"=w442:dbl, "[6]"=w435:dbl, "[7]"=w434:dbl, "[8]"=w433:dbl)
                          n286 = Compound Arithmetic op=ADD(w447, w446, w445, w444, w443, w442) -> (w441:dbl)
                          n287 = Compound Arithmetic op=ADD(w435, w434, w433) -> (w436:dbl)
                          n288 = Bundle(w441) -> (w440:cluster{dbl})  [unwired: 1 in]
                          n289 = Bundle(w436) -> (w437:cluster{dbl})  [unwired: 1 in]
                          n290 = Cluster To Array(cluster=w440) -> (array=w439:dbl[])
                          n291 = Cluster To Array(cluster=w437) -> (array=w438:dbl[])
                          n292 = Byte Array To String(unsigned byte array=w439) -> (string=w431:string)
                          n293 = Byte Array To String(unsigned byte array=w438) -> (string=w432:string)
                          n294 = Concatenate Strings(w431, w432, "CODIGO") -> (w428:string)
                          n295 = local read "Pagina 1"() -> (w426:string)
                          n296 = String Subset(string=w428, offset (0)=0, length (rest)=30 ("length (rest)")) -> (substring=w425:string)
                          n297 = Replace Substring(2:30 ("length (len. of substring)"), 3:225 ("offset (0)"), 4:w425, 5:w426) -> (1:w427:string)  [unwired: 1 out]
                          n298 = local write "Pagina 1"(w427) -> ()
                        }
                        frame #4 {
                          w487 = T21 0 items=["both", "start of string", "end of string"] ("location (both)")
                          n299 = local read "Mapa Ee 492"() -> (w489:string)
                          n300 = local read "Pagina 2"() -> (w498:string)
                          n301 = local read "Pagina 1"() -> (w499:string)
                          n302 = Concatenate Strings(w499, w498) -> (w494:string)
                          n303 = call <vilib>:"Trim Whitespace.vi"("string"=w489, "location (both)"=w487) -> ("trimmed string"=w488:string)
                          n304 = Not Equal?(x=w494, y=w489) -> (x != y?=w497:bool)
                          n305 = Not Equal?(x=w488, y="") -> (x != y?=w495:bool)
                          n306 = local write "Mapa Ee 492"(w494) -> ()
                          n307 = Compound Arithmetic op=AND(w497, w495) -> (w493:bool)
                          "Recup?" <- w493
                          n308 = Select(t=0 ("length (rest)"), s=w493, f=2 ("length (rest)")) -> (s? t:f=w492:i32)
                          n309 = property on="Recuperar" class="Bool (strict)"("Disabled"=w492) -> ()  [unwired: 2 in, 2 out]
                        }
                      }
                      n310 = case shown="True" "Recuperar" {
                        frame False {
                        }
                        frame True {
                          w249 = u16 1 items=["Abrir menu:", "Abrir Archivo", "Guardar Como...", "Leer Eeprom", "Grabar en Eeprom"] ("Manejo de datos:")
                          n311 = local write "Menu 492:"(w249) -> ()
                        }
                      }
                      n312 = property on="Menu 492:" class="Ring (strict)"("Disabled"=u8 0) -> ()  [unwired: 2 in, 2 out]
                      "Menu light" <- TRUE ("Menu light")
                    }
                    frame 1, 3 {
                      n313 = stacked-sequence {
                        tunnel: w503 -> [w520 _ _ _]
                        tunnel: w502 -> [w519 _ _ _]
                        tunnel: w501 -> [w518 _ _ _]
                        tunnel: w500 -> [w517 _ _ _]
                        frame #0 {
                          w509 = u16 0 items=["Abrir menu:", "Abrir Archivo", "Guardar Como...", "Leer Eeprom", "Grabar en Eeprom"] ("Manejo \nde datos:")
                          # "lectura de mapa eeprom o archivo y recuperacion estado ultima session"
                          n314 = case shown="1" w520 {
                            tunnel: [w533 w543] -> w508
                            tunnel: w519 -> [w537 _]
                            tunnel: w518 -> [w536 _]
                            tunnel: w517 -> [w535 _]
                            tunnel: [w538 w542] -> w512
                            frame 3, Default {
                              n315 = call "02lectura_eeprom.vi"("timeout ms"=w535, "puerto"=w536, "Adress"=w537) -> ("error out"=w534:errorcluster, "mapaeeprom"=w533:string, "conn ID"=w532:refnum<k5>)
                              n316 = TCP Close Connection(connection ID=w532) -> ()  [unwired: 1 in, 3 out]
                              n317 = case shown="No Error" w534 {
                                tunnel: [FALSE ("true") w541] -> w538
                                frame No Error {
                                }
                                frame Error {
                                n318 = One Button Dialog(message="ERROR al intentar\nleer memoria Eeprom\n\nPrecione OK para continuar\n" ("y")) -> (true=w541:bool)  [unwired: 1 out]
                                }
                              }
                            }
                            frame 1 {
                              n319 = local read "Recuperar"() -> (w544:bool)
                              n320 = case shown="False" w544 {
                                tunnel: [w548 w556] -> w543
                                tunnel: [w547 w554] -> w542
                                frame False {
                                n321 = Open/Create/Replace File() -> (refnum out=w545:refnum<file>, cancelled=w546:bool)  [unwired: 1 in, 6 out]
                                n322 = case shown="False" w546 {
                                selector: w546 -> [w549 w552]
                                tunnel: [w551 w553] -> w548
                                tunnel: [w549 w552] -> w547
                                tunnel: w545 -> [w550 _]
                                frame False {
                                n323 = Read from Text File(file (use dialog)=w550) -> (text=w551:string)  [unwired: 1 in, 5 out]
                                }
                                frame True {
                                n324 = local read "Mapa Ee 492"() -> (w553:string)
                                }
                                }
                                }
                                frame True {
                                n325 = local write "Recuperar"(FALSE ("Read From File:")) -> ()
                                n326 = Read from Text File() -> (text=w556:string, cancelled=w554:bool)  [unwired: 2 in, 4 out]
                                }
                              }
                            }
                          }
                          n327 = Not Equal?(x="Mapa Ee 492", y=w508) -> (x != y?=w522:bool)
                          n328 = Not Equal?(x="Mapa Ee 492", y="                               \u0000\u0000" ("Mapa Eeprom 2")) -> (x != y?=w516:bool)
                          n329 = Not(x=w512) -> (.not. x?=w510:bool)
                          n330 = Compound Arithmetic op=AND(w516, w522, "Flag write", w510) -> (w521:bool)
                          n331 = case shown="True" w521 {
                            tunnel: [w529 w531] -> w511
                            frame False {
                              w529 = TRUE ("OK Button 2")
                              n332 = local write "Flag write"(w529) -> ()
                            }
                            frame True {
                              n333 = Two Button Dialog(message="La información que desea cargar, difiere a la que\nvisualiza en la pantalla...\n\n\nDesea cargarla de todos modos?") -> (T button?=w531:bool)  [unwired: 2 out]
                            }
                          }
                          n334 = local write "Menu light"(FALSE ("Menu light")) -> ()
                          n335 = Not And(1:w510, 2:w511) -> (0:w507:bool)
                          n336 = property on="Menu 492:" class="Ring (strict)"("Disabled"=u8 2) -> ()  [unwired: 2 in, 2 out]
                          n337 = Select(t="Mapa Ee 492", s=w507, f=w508) -> (s? t:f=w506:string)
                          n338 = local write "Mapa Ee 492"(w506) -> ()
                          n339 = String Subset(string=w506, offset (0)=0, length (rest)=256 ("length (rest)")) -> (substring=→"Pagina 1":string)
                          n340 = String Subset(string=w506, offset (0)=256, length (rest)=256 ("length (rest)")) -> (substring=→"Pagina 2":string)
                          n341 = local write "Menu 492:"(w509) -> ()
                        }
                        frame #1 {
                          w557 = T21 2 items=["both", "start of string", "end of string"] ("location (both)")
                          # "Se adquieren los primeros 33 bytes de la pag0 y los nombres de las señales logicas en pag1"
                          n342 = local read "Mapa Ee 492"() -> (w566:string)
                          n343 = String Subset(string=w566, offset (0)=225, length (rest)=1 ("length (rest)")) -> (substring=w586:string)
                          n344 = String Subset(string=w566, offset (0)=226, length (rest)=1 ("length (rest)")) -> (substring=w567:string)
                          n345 = String Subset(string=w566, offset (0)=227, length (rest)=28 ("length (rest)")) -> (substring=w565:string)
                          n346 = String Subset(string=w566, offset (0)=31, length (rest)=1 ("length (rest)")) -> (substring=w570:string)
                          n347 = String Subset(string=w566, offset (0)=32, length (rest)=1 ("length (rest)")) -> (substring=w588:string)
                          n348 = String Subset(string=w566, offset (0)=8, length (rest)=23 ("length (rest)")) -> (substring=w559:string)
                          n349 = String Subset(string=w566, offset (0)=0, length (rest)=8 ("length (rest)")) -> (substring=w560:string)
                          n350 = String To Byte Array(string=w586) -> (unsigned byte array=w583:u8[])
                          n351 = String To Byte Array(string=w567) -> (unsigned byte array=w577:u8[])
                          n352 = String To Byte Array(string=w588) -> (unsigned byte array=w590:u8[])
                          n353 = String To Byte Array(string=w570) -> (unsigned byte array=w573:u8[])
                          n354 = call <vilib>:"Trim Whitespace.vi"("string"=w560, "location (both)"=w557) -> ("trimmed string"=w561:string)
                          n355 = Array To Cluster(array=w583) -> (cluster=w582:cluster{"unsigned byte array[0]":u8})
                          n356 = Array To Cluster(array=w577) -> (cluster=w578:cluster{"unsigned byte array[0]":u8})
                          n357 = local write "CODIGO"(w565) -> ()
                          n358 = call <vilib>:"Trim Whitespace.vi"("string"=w559, "location (both)"=w557) -> ("trimmed string"=w558:string)
                          n359 = Array To Cluster(array=w590) -> (cluster=w589:cluster{"unsigned byte array[0]":u8})
                          n360 = Array To Cluster(array=w573) -> (cluster=w572:cluster{"unsigned byte array[0]":u8})
                          n361 = Unbundle(w582) -> ("unsigned byte array[0]"=w581:u8)
                          n362 = Unbundle(w578) -> ("unsigned byte array[0]"=w576:u8)
                          n363 = local write "Rotulo izquierdo:"(w561) -> ()
                          n364 = local write "Rotulo derecho:"(w558) -> ()
                          n365 = Unbundle(w589) -> ("unsigned byte array[0]"=w563:u8)
                          n366 = Unbundle(w572) -> ("unsigned byte array[0]"=w571:u8)
                          n367 = local write "Medición Ampliada:"(w563) -> ()
                          n368 = expression code="(x+1)*4"(w571) -> (w564:u8)
                          n369 = for {
                            N: 9 -> [_]
                            tunnel: [w612] -> w562 mode=indexing
                            tunnel: w581 -> [w604]
                            tunnel: w576 -> [w601]
                            tunnel: w566 -> [w600]
                            i -> [w607]
                            w597 = T21 2 items=["both", "start of string", "end of string"] ("location (both)")
                            n370 = case shown="6..8" w607 {
                              selector: w607 -> [w616 w619]
                              tunnel: [w616 w618] -> w606
                              tunnel: w604 -> [w615 _]
                              tunnel: [w615 w620] -> w603
                              tunnel: w601 -> [_ w620]
                              frame 0, Default {
                              }
                              frame 6..8 {
                                n371 = Subtract(x=w619, y=6) -> (x-y=w618:i32)
                              }
                            }
                            n372 = expression code="14*32+(x*7)"(w607) -> (w613:i32)
                            n373 = Increment(x=w607) -> (x+1=w611:i32)
                            n374 = Scale By Power Of 2(n=w606, x=1.0) -> (x*2^n=w605:dbl)
                            n375 = String Subset(string=w600, offset (0)=w613, length (rest)=7 ("length (rest)")) -> (substring=w598:string)
                            n376 = And(x=w605, y=w603) -> (x .and. y?=w602:i32)
                            n377 = call <vilib>:"Trim Whitespace.vi"("string"=w598, "location (both)"=w597) -> ("trimmed string"=w599:string)
                            n378 = Not Equal To 0?(x=w602) -> (x != 0?=w609:bool)
                            n379 = Bundle(w611, "trimmed string"=w599, w609) -> (w610:cluster{i32, "trimmed string":string, bool})  [unwired: 1 out]
                            n380 = Build Array(w610) -> (w612:cluster{i32, "trimmed string":string, bool}[])
                          }
                          n381 = local write "Cant Med:"(w564) -> ()
                          n382 = local write "Señales Logicas:"(w562) -> ()
                        }
                        frame #2 {
                          # "Datos de las mediciones de la pagina0"
                          n383 = local read "Pagina 1"() -> (w626:string)
                          n384 = for {
                            N: 16 -> [_]
                            tunnel: [w655] -> w625 mode=indexing
                            tunnel: w626 -> [w641]
                            i -> [w643]
                            w636 = T21 2 items=["both", "start of string", "end of string"] ("location (both)")
                            n385 = expression code="33+(x*12)"(w643) -> (w648:i32)
                            n386 = Add(x=w648, y=11) -> (x+y=w650:i32)
                            n387 = Add(x=w648, y=10) -> (x+y=w671:i32)
                            n388 = Add(x=w648, y=7) -> (x+y=w670:i32)
                            n389 = String Subset(string=w641, offset (0)=w650, length (rest)=1 ("length (rest)")) -> (substring=w645:string)
                            n390 = String Subset(string=w641, offset (0)=w671, length (rest)=1 ("length (rest)")) -> (substring=w662:string)
                            n391 = String Subset(string=w641, offset (0)=w648, length (rest)=7 ("length (rest)")) -> (substring=w639:string)
                            n392 = String Subset(string=w641, offset (0)=w670, length (rest)=3 ("length (rest)")) -> (substring=w640:string)
                            n393 = String To Byte Array(string=w645) -> (unsigned byte array=w647:u8[])
                            n394 = call <vilib>:"Trim Whitespace.vi"("string"=w639, "location (both)"=w636) -> ("trimmed string"=w638:string)
                            n395 = String To Byte Array(string=w662) -> (unsigned byte array=w667:u8[])
                            n396 = String To Byte Array(string=w662) -> (unsigned byte array=w664:u8[])
                            n397 = Array To Cluster(array=w647) -> (cluster=w646:cluster{"unsigned byte array[0]":u8})
                            n398 = Array To Cluster(array=w667) -> (cluster=w666:cluster{"unsigned byte array[0]":u8})
                            n399 = Array To Cluster(array=w664) -> (cluster=w665:cluster{"unsigned byte array[0]":u8})
                            n400 = call <vilib>:"Trim Whitespace.vi"("string"=w640, "location (both)"=w636) -> ("trimmed string"=w637:string)
                            n401 = Increment(x=w643) -> (x+1=w642:i32)
                            n402 = Unbundle(w646) -> ("unsigned byte array[0]"=w644:u8)
                            n403 = Unbundle(w666) -> ("unsigned byte array[0]"=w659:u8)
                            n404 = Unbundle(w665) -> ("unsigned byte array[0]"=w661:u8)
                            n405 = Compound Arithmetic op=AND(w659, u8 240 ("value")) -> (w657:u8)
                            n406 = Compound Arithmetic op=AND(w661, u8 15 ("value")) -> (w652:u8)
                            n407 = Divide(x=w657, y=u8 16) -> (x/y=w654:dbl)
                            n408 = To Unsigned Byte Integer(number=w652) -> (unsigned 8bit integer=w653:u8)
                            n409 = Bundle(w642, "trimmed string"=w638, "trimmed string"=w637, w654, w653, "unsigned byte array[0]"=w644) -> (w656:T28)  [unwired: 1 out]
                            n410 = Build Array(w656) -> (w655:T29)
                          }
                          n411 = Array Subset(array=w625, index (row)=0 ("index"), length (row)=4 ("length")) -> (w624:T30)  [unwired: 2 in]
                          n412 = Array Subset(array=w625, index (row)=4 ("index"), length (row)=4 ("length")) -> (w623:T30)  [unwired: 2 in]
                          n413 = Array Subset(array=w625, index (row)=8 ("index"), length (row)=4 ("length")) -> (w622:T30)  [unwired: 2 in]
                          n414 = Array Subset(array=w625, index (row)=12 ("index"), length (row)=4 ("length")) -> (w621:T30)  [unwired: 2 in]
                          n415 = local write "ARRAY 1"(w625) -> ()
                          n416 = local write "Med 13-16"(w621) -> ()
                          n417 = local write "Med 1-4"(w624) -> ()
                          n418 = local write "Med 9-12"(w622) -> ()
                          n419 = local write "Med 5-8"(w623) -> ()
                        }
                        frame #3 {
                          # "Datos de las mediciones de la pagina1"
                          n420 = local read "Pagina 2"() -> (w680:string)
                          n421 = for {
                            N: 16 -> [_]
                            tunnel: [w710] -> w679 mode=indexing
                            tunnel: w680 -> [w695]
                            i -> [w697]
                            w690 = T21 2 items=["both", "start of string", "end of string"] ("location (both)")
                            n422 = expression code="x*12"(w697) -> (w703:i32)
                            n423 = Add(x=w703, y=7) -> (x+y=w725:i32)
                            n424 = Add(x=w703, y=10) -> (x+y=w726:i32)
                            n425 = Add(x=w703, y=11) -> (x+y=w705:i32)
                            n426 = String Subset(string=w695, offset (0)=w726, length (rest)=1 ("length (rest)")) -> (substring=w717:string)
                            n427 = String Subset(string=w695, offset (0)=w703, length (rest)=7 ("length (rest)")) -> (substring=w694:string)
                            n428 = String Subset(string=w695, offset (0)=w725, length (rest)=3 ("length (rest)")) -> (substring=w692:string)
                            n429 = String Subset(string=w695, offset (0)=w705, length (rest)=1 ("length (rest)")) -> (substring=w700:string)
                            n430 = String To Byte Array(string=w717) -> (unsigned byte array=w722:u8[])
                            n431 = String To Byte Array(string=w717) -> (unsigned byte array=w719:u8[])
                            n432 = String To Byte Array(string=w700) -> (unsigned byte array=w702:u8[])
                            n433 = Array To Cluster(array=w722) -> (cluster=w721:cluster{"unsigned byte array[0]":u8})
                            n434 = Array To Cluster(array=w719) -> (cluster=w720:cluster{"unsigned byte array[0]":u8})
                            n435 = call <vilib>:"Trim Whitespace.vi"("string"=w694, "location (both)"=w690) -> ("trimmed string"=w693:string)
                            n436 = Array To Cluster(array=w702) -> (cluster=w701:cluster{"unsigned byte array[0]":u8})
                            n437 = Unbundle(w721) -> ("unsigned byte array[0]"=w714:u8)
                            n438 = Unbundle(w720) -> ("unsigned byte array[0]"=w716:u8)
                            n439 = call <vilib>:"Trim Whitespace.vi"("string"=w692, "location (both)"=w690) -> ("trimmed string"=w691:string)
                            n440 = Unbundle(w701) -> ("unsigned byte array[0]"=w699:u8)
                            n441 = Compound Arithmetic op=AND(w716, u8 15 ("value")) -> (w707:u8)
                            n442 = Compound Arithmetic op=AND(w714, u8 240 ("value")) -> (w712:u8)
                            n443 = To Unsigned Byte Integer(number=w707) -> (unsigned 8bit integer=w708:u8)
                            n444 = Add(x=w697, y=17) -> (x+y=w698:i32)
                            n445 = Divide(x=w712, y=u8 16) -> (x/y=w709:dbl)
                            n446 = Bundle(w698, "trimmed string"=w693, "trimmed string"=w691, w709, w708, "unsigned byte array[0]"=w699) -> (w711:T28)  [unwired: 1 out]
                            n447 = Build Array(w711) -> (w710:T29)
                          }
                          n448 = Array Subset(array=w679, index (row)=0 ("index"), length (row)=4 ("length")) -> (w677:T30)  [unwired: 2 in]
                          n449 = Array Subset(array=w679, index (row)=4 ("index"), length (row)=4 ("length")) -> (w678:T30)  [unwired: 2 in]
                          n450 = Array Subset(array=w679, index (row)=8 ("index"), length (row)=4 ("length")) -> (w676:T30)  [unwired: 2 in]
                          n451 = Array Subset(array=w679, index (row)=12 ("index"), length (row)=4 ("length")) -> (w675:T30)  [unwired: 2 in]
                          n452 = local write "ARRAY 2"(w679) -> ()
                          n453 = local write "Med 17-20"(w677) -> ()
                          n454 = local write "Med 21-24"(w678) -> ()
                          n455 = local write "Med 25-28"(w676) -> ()
                          n456 = local write "Med 29-32"(w675) -> ()
                        }
                      }
                    }
                    frame 2 {
                      w737 = u16 0 items=["Abrir menu:", "Abrir Archivo", "Guardar Como...", "Leer Eeprom", "Grabar en Eeprom"] ("Manejo \nde datos:")
                      # "SE GUARDA MAPA EEPROM EN ARCHIVO"
                      n457 = local read "Mapa Ee 492"() -> (w738:string)
                      n458 = local write "Menu light"(FALSE ("Menu light")) -> ()
                      n459 = local write "Menu 492:"(w737) -> ()
                      n460 = Write to Text File(text=w738) -> (cancelled=w734:bool, error out=w732:errorcluster)  [unwired: 2 in, 2 out]
                      n461 = Unbundle(w732) -> ("status"=w731:bool)  [unwired: 2 out]
                      n462 = Not(x=w731) -> (.not. x?=w730:bool)
                      n463 = property on="Menu 492:" class="Ring (strict)"("Disabled"=u8 2) -> ()  [unwired: 2 in, 2 out]
                      n464 = Or(x=w734, y=w730) -> (x .or. y?=w733:bool)
                      n465 = case shown="False" w733 {
                        frame False {
                          n466 = One Button Dialog(message="Error al escribir en archivo...\n\nPrecione OK para continuar") -> ()  [unwired: 2 out]
                        }
                        frame True {
                        }
                      }
                    }
                    frame 4 {
                      # "GRABA MAPAEEPROM EN MEMORIA DEL EQUIPO"
                      # "permite la carga sin preguntas\nde lectura eeprom despues de grabarla"
                      n467 = local read "Pagina 1"() -> (w741:string)
                      n468 = local read "Pagina 2"() -> (w740:string)
                      n469 = call "02grabareeprom.vi"("Pagina 2"=w740, "Pagina 1"=w741, "timeout ms (500)"=w748, "Puerto"=w747, "address"=w746) -> ("Error?"=w742:bool)
                      n470 = case shown="False" w742 {
                        frame False {
                          w749 = u16 3 items=["Abrir menu:", "Abrir Archivo", "Guardar Como...", "Leer Eeprom", "Grabar en Eeprom"] ("Manejo \nde datos:")
                          n471 = local read "Equipo Nº"() -> (w751:i32)
                          n472 = local read "EE 492 in"() -> (w750:T5)
                          n473 = local read "Pagina 1"() -> (w756:string)
                          n474 = local read "Pagina 2"() -> (w755:string)
                          n475 = Index Array(array=w750, index=w751) -> (element=w761:T31)
                          n476 = Concatenate Strings(w756, w755) -> (w754:string)
                          n477 = Unbundle(w761) -> ("cantmedic"=w757:u8, "Med_nom"=w758:string[], "Med_unid"=w759:string[], "Med_caract"=w760:string)  [unwired: 1 out]
                          n478 = Bundle(w754, "cantmedic"=w757, "Med_nom"=w758, "Med_unid"=w759, "Med_caract"=w760) -> (w753:T32)  [unwired: 1 out]
                          n479 = Replace Array Subset(array=w750, new element=w753, index=w751) -> (w752:T5)
                          n480 = local write "Menu 492:"(w749) -> ()
                          n481 = local write "EE 492 in"(w752) -> ()
                        }
                        frame True {
                          w763 = u16 0 items=["Abrir menu:", "Abrir Archivo", "Guardar Como...", "Leer Eeprom", "Grabar en Eeprom"] ("Manejo \nde datos:")
                          n482 = local write "Menu 492:"(w763) -> ()
                          n483 = One Button Dialog(message="Error al escribir Eeprom...\n\nPrecione OK para continuar") -> ()  [unwired: 2 out]
                        }
                      }
                      n484 = local write "Menu light"(FALSE ("Menu light")) -> ()
                      n485 = local write "Flag write"(FALSE ("Flag write")) -> ()
                      n486 = property on="Menu 492:" class="Ring (strict)"("Disabled"=u8 2) -> ()  [unwired: 2 in, 2 out]
                    }
                    frame 5 {
                      w764 = u16 0 items=["   Menu:"=0, "_______________"=100, "Abrir Archivo"=1, "Guardar Como..."=2, "_______________"=200, "Leer Eeprom"=3, "Grabar en Eeprom"=4, "_______________"=300, "Exit"=5] ("Manejo \nde datos:")
                      # "EXIT! desde el menu"
                      n487 = local write "Menu 492:"(w764) -> ()
                      n488 = local write "Stop"(TRUE ("Stop")) -> ()
                    }
                    frame 6 {
                      w766 = 0
                      w768 = u16 0 items=["Abrir menu:", "Abrir Archivo", "Guardar Como...", "Leer Eeprom", "Grabar en Eeprom"] ("Manejo \nde datos:")
                      w771 = "" ("Rotulo1:")
                      # "RESET MAPA"
                      n489 = for {
                        N: 9 -> [_]
                        tunnel: [w793] -> w769 mode=indexing
                        i -> [w792]
                        n490 = Increment(x=w792) -> (x+1=w791:i32)
                        n491 = Bundle(w791, "mapaeeprom"="", TRUE) -> (w794:cluster{i32, "mapaeeprom":string, bool})  [unwired: 1 out]
                        n492 = Build Array(w794) -> (w793:cluster{i32, "mapaeeprom":string, bool}[])
                      }
                      n493 = for {
                        N: 8 -> [_]
                        i -> [w773]
                        n494 = expression code="X*4+1"(w773) -> (w772:i32)
                        n495 = for {
                          N: 4 -> [_]
                          tunnel: [w789] -> w774 mode=indexing
                          tunnel: w772 -> [w786]
                          i -> [w787]
                          w785 = 0
                          w784 = "" ("mapaeeprom")
                          n496 = Add(x=w786, y=w787) -> (x+y=w788:i32)
                          n497 = Bundle(w788, "mapaeeprom"=w784, "mapaeeprom"=w784, w785, w785, w785) -> (w790:T33)  [unwired: 1 out]
                          n498 = Build Array(w790) -> (w789:T34)
                        }
                        n499 = case shown="6" w773 {
                          tunnel: w774 -> [w776 w777 w778 w779 w780 w781 w782 w783]
                          frame 0, Default {
                            n500 = local write "Med 1-4"(w776) -> ()
                          }
                          frame 1 {
                            n501 = local write "Med 5-8"(w777) -> ()
                          }
                          frame 2 {
                            n502 = local write "Med 9-12"(w778) -> ()
                          }
                          frame 3 {
                            n503 = local write "Med 13-16"(w779) -> ()
                          }
                          frame 4 {
                            n504 = local write "Med 17-20"(w780) -> ()
                          }
                          frame 5 {
                            n505 = local write "Med 21-24"(w781) -> ()
                          }
                          frame 6 {
                            n506 = local write "Med 25-28"(w782) -> ()
                          }
                          frame 7 {
                            n507 = local write "Med 29-32"(w783) -> ()
                          }
                        }
                      }
                      n508 = local write "Señales Logicas:"(w769) -> ()
                      n509 = call "Time Delay3"() -> ()  [unwired: 2 in, 10 out]
                      n510 = local write "Rotulo izquierdo:"(w771) -> ()
                      n511 = local write "Rotulo derecho:"(w771) -> ()
                      n512 = local write "Menu 492:"(w768) -> ()
                      n513 = local write "Medición Ampliada:"(w766) -> ()
                      n514 = local write "Cant Med:"(w766) -> ()
                    }
                  }
                }
                frame "568" {
                  w800 = u8 0 items=["Equipo Nº 01", "Equipo Nº 02", "Equipo Nº 03", "Equipo Nº 04", "Equipo Nº 05", "Equipo Nº 06", "Equipo Nº 07", "Equipo Nº 08"] ("Equipo Nº")
                  w813 = u8 6 items=["   Menu:"=0, "_______________"=101, "Abrir Archivo"=1, "Guardar Como..."=2, "_______________"=102, "Leer Memoria"=3, "Grabar Memoria"=4, "_______________"=103, "Reset Panel"=6] ("Menu:")
                  n515 = Bundle("IP"=w804, "Puerto:"=w803, "Time Out"=w802) -> (w801:T35)  [unwired: 1 in]
                  n516 = feedback #3(u8 4 ("Equipo Nº")) -> (w806:u8)
                  n517 = feedback #4(w813) -> (w812:u8)
                  n518 = feedback-in #4("Menu 568:") -> ()
                  n519 = Not Equal?(x="Menu 568:", y=w812) -> (x != y?=w814:bool)
                  n520 = Not Equal?(x=w812, y=w813) -> (x != y?=w811:bool)
                  n521 = Select(t="Slave Nº", s="MASTER\n/SLAVE", f=w800) -> (s? t:f=w798:u8)
                  n522 = feedback-in #3(w798) -> ()
                  n523 = Not Equal?(x=w798, y=w806) -> (x != y?=w805:bool)
                  n524 = Select(t=w814, s=w811, f=FALSE) -> (s? t:f=w810:bool)
                  n525 = property on="Slave Nº" class="Ring (strict)"("Visible"="MASTER\n/SLAVE") -> ()  [unwired: 2 in, 2 out]
                  n526 = Or(x=w810, y=w805) -> (x .or. y?=w807:bool)
                  n527 = case shown="5" "Menu 568:" {
                    selector: "Menu 568:" -> [_ w847 w898 _ _]
                    tunnel: w798 -> [w816 w846 w897 _ _]
                    tunnel: w807 -> [w817 _ _ _ _]
                    tunnel: w801 -> [_ w845 w892 _ _]
                    tunnel: w798 -> [_ w844 _ _ _]
                    frame 0, Default {
                      n528 = local read "Cantidad\nMediciones"() -> (w821:u8)
                      n529 = case shown="True" w817 {
                        tunnel: w816 -> [_ w831]
                        frame False {
                        }
                        frame True {
                          # "DECODIFICA PARA MOSTRAR EN PANTALLA"
                          n530 = case shown="0" w831 {
                            tunnel: [w842 w843] -> w832
                            frame 1, Default {
                              n531 = local read "Eeprom D-cod S"() -> (w842:T1)
                            }
                            frame 0 {
                              n532 = local read "Eeprom D-cod M"() -> (w843:T1)
                            }
                          }
                          n533 = Unbundle(w832) -> ("Rotulo 1"=w840:string, "Rotulo 2"=w839:string, "Cant. Meds."=w833:u8, "Med ampl"=w841:u8, "Analogicas 16"=w838:T36, "Analogicas 32"=w837:T37, "DIG_8"=w836:T13, "DIG_16"=w835:T13, "PWM"=w834:T15)
                          n534 = local write "Cantidad\nMediciones"(w833) -> ()
                          n535 = local write "Medición Ampliada: 2"(w841) -> ()
                          n536 = local write "Título Secundario:"(w839) -> ()
                          n537 = local write "Título Principal:"(w840) -> ()
                          n538 = local write "PWM data 1&2"(w834) -> ()
                          n539 = local write "DIG_16"(w835) -> ()
                          n540 = local write "Ana 16"(w838) -> ()
                          n541 = local write "Ana 32"(w837) -> ()
                          n542 = local write "DIG_8"(w836) -> ()
                        }
                      }
                      n543 = Less?(x=w821, y=u8 17) -> (x < y?=w828:bool)
                      n544 = Decrement(x=w821) -> (x-1=w830:u8)
                      n545 = Less?(x=w821, y=u8 1) -> (x < y?=w823:bool)
                      n546 = Boolean To (0,1)(Boolean=w828) -> (0, 1=w827:i16)
                      n547 = Boolean To (0,1)(Boolean=w823) -> (0, 1=w824:i16)
                      n548 = property on="Medición Ampliada: 2" class="Ring (strict)"("Maximum"=w830) -> ()  [unwired: 2 in, 2 out]
                      n549 = Multiply(x=w827, y=i16 2) -> (x*y=w818:i16)
                      n550 = Multiply(x=w824, y=i16 2) -> (x*y=w820:i16)
                      n551 = property on="Ana 16" class="Arr (strict)"("DisabledEnum"=w820) -> ()  [unwired: 2 in, 2 out]
                      n552 = property on="Ana 32" class="Arr (strict)"("DisabledEnum"=w818) -> ()  [unwired: 2 in, 2 out]
                      n553 = call "Time Delay"() -> ()  [unwired: 11 in, 1 out]
                      "Menu light 2" <- TRUE ("Menu light")
                    }
                    frame 2, 4 {
                      n554 = stacked-sequence {
                        tunnel: w847 -> [_ w871]
                        tunnel: w846 -> [_ w870]
                        tunnel: w845 -> [_ w869]
                        tunnel: w844 -> [w850 _]
                        frame #0 {
                          # "RECODIFICA EL MAPA EEPROM"
                          n555 = call "eeprom-recode.vi"("PWM"="PWM data 1&2", "Rotulo izquierdo:"="Título Principal:", "Rotulo derecho:"="Título Secundario:", "Cant Med:"="Cantidad\nMediciones", "Medición Ampliada:"="Medición Ampliada: 2", "DIG_16"="DIG_16", "DIG_8"="DIG_8", "Ana 32"="Ana 32", "Ana 16"="Ana 16") -> ("Recoded eeprom"=w849:string)
                          "eeprom re-cod" <- w849
                          n556 = local write "Menu light 2"(FALSE ("Menu light")) -> ()
                          n557 = call "deco_ee_568.vi"("data IN"=w849) -> ("Eeprom"=w848:T38)  [unwired: 2 in, 2 out]
                          n558 = case shown="3, 5, 7, 9, 11, 13, 15, Default" w850 {
                            selector: w850 -> [w861 _]
                            tunnel: w848 -> [w863 w865]
                            frame 3, 5, 7, 9, 11, 13, 15, Default {
                              n559 = local read "EE 568 S IN"() -> (w862:T2)
                              n560 = Replace Array Subset(array=w862, new element=w863, index=w861) -> (w864:T2)
                              n561 = local write "EE 568 S IN"(w864) -> ()
                            }
                            frame 1 {
                              n562 = local read "EE 568 M IN"() -> (w867:T2)
                              n563 = local read "Equipo Nº"() -> (w868:i32)
                              n564 = Replace Array Subset(array=w867, new element=w865, index=w868) -> (w866:T2)
                              n565 = local write "EE 568 M IN"(w866) -> ()
                            }
                          }
                        }
                        frame #1 {
                          # "ESCRIBE EEPROM"
                          n566 = case shown="4" w871 {
                            tunnel: w870 -> [_ w881]
                            tunnel: w869 -> [_ w880]
                            frame 2, Default {
                              w872 = u8 0 items=["   Menu:"=0, "_______________"=101, "Abrir Archivo"=1, "Guardar Como..."=2, "_______________"=102, "Leer Memoria"=3, "Grabar Memoria"=4, "_______________"=103, "Reset Panel"=6, "_______________"=104, "Salir"=5] ("Menu:")
                              # "ESCRIBE EEPROM A ARCHIVO"
                              n567 = local read "eeprom re-cod"() -> (w873:string)
                              n568 = local write "Menu 568:"(w872) -> ()
                              n569 = Write to Text File(text=w873) -> (cancelled=w874:bool, error out=w876:errorcluster)  [unwired: 2 in, 2 out]
                              n570 = Unbundle(w876) -> ("status"=w877:bool)  [unwired: 2 out]
                              n571 = Not(x=w877) -> (.not. x?=w878:bool)
                              n572 = Or(x=w874, y=w878) -> (x .or. y?=w875:bool)
                              n573 = case shown="False" w875 {
                                frame False {
                                n574 = One Button Dialog(message="No se ha guardado en archivo...\n\nPrecione OK para continuar") -> ()  [unwired: 2 out]
                                }
                                frame True {
                                }
                              }
                            }
                            frame 4 {
                              # "ESCRIBE EEPROM EN PLACA"
                              n575 = local read "eeprom re-cod"() -> (w883:string)
                              n576 = Concatenate Strings(w883, "                             " ("string")) -> (w885:string)
                              n577 = String Subset(string=w885, length (rest)=550 ("length (rest)")) -> (substring=w882:string)  [unwired: 1 in]
                              n578 = call "graba-eeprom.vi"("Equipo Nº"=w881, "Eeprom"=w882, "COM DATA"=w880) -> ("error out"=w889:errorcluster)  [unwired: 3 in]
                              n579 = Unbundle(w889) -> ("status"=w888:bool)  [unwired: 2 out]
                              n580 = local write "COMFAIL M"(w888) -> ()
                              n581 = case shown="False" w888 {
                                tunnel: [w890 w891] -> w887
                                frame False {
                                w890 = u8 3 items=["   Menu:"=0, "_______________"=101, "Abrir Archivo"=1, "Guardar Como..."=2, "_______________"=102, "Leer Memoria"=3, "Grabar Memoria"=4, "_______________"=103, "Reset Panel"=6, "_______________"=104, "Salir"=5] ("Menu:")
                                n582 = call "Time 0,"() -> ()  [unwired: 11 in, 1 out]
                                }
                                frame True {
                                w891 = u8 0 items=["   Menu:"=0, "_______________"=101, "Abrir Archivo"=1, "Guardar Como..."=2, "_______________"=102, "Leer Memoria"=3, "Grabar Memoria"=4, "_______________"=103, "Reset Panel"=6, "_______________"=104, "Salir"=5] ("Menu:")
                                }
                              }
                              n583 = local write "Menu 568:"(w887) -> ()
                            }
                          }
                        }
                      }
                    }
                    frame 1, 3 {
                      w896 = u8 0 items=["   Menu:"=0, "_______________"=101, "Abrir Archivo"=1, "Guardar Como..."=2, "_______________"=102, "Leer Memoria"=3, "Grabar Memoria"=4, "_______________"=103, "Reset Panel"=6, "_______________"=104, "Salir"=5] ("Menu:")
                      # "LECTURA DE MAPA EEPROM"
                      n584 = case shown="3" w898 {
                        tunnel: [w901 w911] -> w895
                        tunnel: w897 -> [_ w910]
                        tunnel: w892 -> [_ w909]
                        frame 1, Default {
                          # "CARGAR DESDE ARCHIVO"
                          n585 = Open/Create/Replace File() -> (refnum out=w903:refnum<file>, cancelled=w904:bool, error out=w902:errorcluster)  [unwired: 1 in, 5 out]
                          n586 = local write "error out"(w902) -> ()
                          n587 = case shown="False" w904 {
                            tunnel: w903 -> [w906 _]
                            tunnel: [w905 w907] -> w901
                            frame False {
                              n588 = Read from Text File(file (use dialog)=w906) -> (text=w905:string)  [unwired: 1 in, 5 out]
                            }
                            frame True {
                              n589 = local read "eeprom re-cod"() -> (w907:string)
                            }
                          }
                        }
                        frame 3 {
                          # "LEE EEPROM DESDE PLACA"
                          n590 = call "lee-eeprom.vi"("Equipo Nº"=w910, "COM DATA"=w909) -> ("COM FAIL"=→"COMFAIL M":bool, "LECTURA"=w911:string, "error out"=w912:errorcluster)  [unwired: 1 in, 1 out]
                          n591 = Unbundle(w912) -> ()  [unwired: 3 out]
                        }
                      }
                      n592 = call "deco_ee_568.vi"("data IN"=w895) -> ("Eeprom"=w893:T38)  [unwired: 2 in, 2 out]
                      n593 = case shown="0" w897 {
                        tunnel: w893 -> [w899 w900]
                        frame 1, Default {
                          n594 = local write "Eeprom D-cod S"(w899) -> ()
                        }
                        frame 0 {
                          n595 = local write "Eeprom D-cod M"(w900) -> ()
                        }
                      }
                      n596 = local write "Menu light 2"(FALSE ("Menu light")) -> ()
                      n597 = local write "Menu 568:"(w896) -> ()
                    }
                    frame 5 {
                      w913 = u16 0 items=["   Menu:"=0, "_______________"=100, "Abrir Archivo"=1, "Guardar Como..."=2, "_______________"=200, "Leer Eeprom"=3, "Grabar en Eeprom"=4, "_______________"=300, "Exit"=5] ("Manejo \nde datos:")
                      n598 = local write "Menu 492:"(w913) -> ()
                      n599 = local write "Stop"(TRUE ("Stop")) -> ()
                    }
                    frame 6 {
                      w917 = T13 [] ("DIG_8")
                      w918 = u8 0 items=["0"=0, "4"=4, "8"=8, "12"=12, "16"=16, "20"=20, "24"=24, "28"=28, "32"=32, "36"=36, "40"=40, "44"=44, "48"=48, "52"=52, "56"=56, "60"=60, "64"=64] ("Cant Med:")
                      w919 = u8 0 items=["   Menu:"=0, "_______________"=101, "Abrir Archivo"=1, "Guardar Como..."=2, "_______________"=102, "Leer Memoria"=3, "Grabar Memoria"=4, "_______________"=103, "Reset Panel"=6] ("Menu:")
                      w920 = u8 0 items=["1", "2", "3", "4", "5", "6", "7", "8", "9", "10", "11", "12", "13", "14", "15", "16", "17", "18", "19", "20", "21", "22", "23", "24", "25", "26", "27", "28", "29", "30", "31", "32", "33", "34", "35", "36", "37", "38", "39", "40", "41", "42", "43", "44", "45", "46", "47", "48", "49", "50", "51", "52", "53", "54", "55", "56", "57", "58", "59", "60", "61", "62", "63", "64"] ("Medición Ampliada:")
                      w921 = "" ("Rotulo izquierdo:")
                      w922 = T39 [] ("Ana 16")
                      # "RESET DE PANEL"
                      n600 = local write "Cantidad\nMediciones"(w918) -> ()
                      n601 = local write "Medición Ampliada: 2"(w920) -> ()
                      n602 = local write "Título Principal:"(w921) -> ()
                      n603 = local write "Título Secundario:"(w921) -> ()
                      n604 = local write "Ana 16"(w922) -> ()
                      n605 = local write "Ana 32"(w922) -> ()
                      n606 = local write "Menu light 2"(FALSE ("Menu light")) -> ()
                      n607 = local write "PWM data 1&2"(T15 {"CONF_PWM1"=0, "VALOR_PWM1"=0, "CONF_PWM2"=0, "VALOR_PWM2"=0} ("PWM")) -> ()
                      n608 = local write "Menu 568:"(w919) -> ()
                      n609 = local write "DIG_8"(w917) -> ()
                      n610 = local write "DIG_16"(w917) -> ()
                    }
                  }
                }
              }
              n611 = Not Equal?(x=w239, y=w240) -> (x != y?=w237:bool)
              n612 = Compound Arithmetic op=OR(w237, "Stop") -> (w241:bool)
            }
          }
        }
      }
    }
    frame #2 {
      n613 = local read "Paneles in"() -> (→"Paneles out":T4)
      n614 = local write "Stop"(FALSE ("Stop")) -> ()
      "EE 492 OUT" <- "EE 492 in"
      "EE 568 M OUT" <- "EE 568 M IN"
      "EE 568 S OUT" <- "EE 568 S IN"
    }
  }
